vi "MainPr(Calculation)-40.vi"() -> ()   [LabVIEW 2013]
doc: "Main Program for Tracking\nThis VI Represents Front Panel and Control Buttons for Perform Tracking\nPlease, optimize the front panel for your own monitor resolution and needs"
uses:
  <vilib>/vision/Avi.llb/IMAQ AVI2 Refnum.ctl
  <vilib>/vision/NI_Vision_Development_Module.lvlib
panel:
  out "error out":errorcluster
  in  "STOP Program":bool
  in  "Front Panel":T1(tab)
  in  "FrameCtl":u32 max=299
  out "1st Movie (Comparison)":T2(plugin-control)
  out "1st Movie":T2(plugin-control)
  in  "Gamma":sgl format="%.2f"
  in  "Operator G Correction":T3(ring)
  in  "Parameter LoG":sgl format="%.2f"
  in  "Operator LoG":T3(ring)
  in  "1/2 Channels":bool
  in  "Sigma":dbl min=0.1
  in  "FrameCtl2":u32 max=499
  in  "Gray or Binarized?":bool
  out "1st Movie Original":T2(plugin-control)
  out "1st Movie Processed":T2(plugin-control)
  in  "Index for thresholding":i8 min=-9
  in  "Keep Nega-\ntive Values?":bool
  out "Detection Progress":u8(slide) scale=0.0..100.0
  in  "# of Frame":u32 max=499
  in  "Save pics (ex)":bool
  in  "Find ALL objects":bool
  out "Results on 1st Movie":T2(plugin-control)
  out "1st Filtering":T2(plugin-control)
  in  "Try my filters!":bool
  in  "# Erosion":i32=2
  in  "Connectivity":bool=TRUE
  in  "Min  Diam":dbl
  in  "Max  Diam":dbl min=12.0
  in  "Filter Tracks":bool
  out "Tracking progress":u8(slide) scale=0.0..100.0
  in  "Save pictures":bool
  in  "Save movies":bool
  in  "Frame":u32 max=499
  in  "Delete Tracs":bool
  out "1st Filtered":T2(plugin-control)
  in  "dR max":dbl min=1.0
  out "1st Filtering (NN)":T2(plugin-control)
  in  "dR min":dbl min=0.0 max=10.0
  out "Raw #":i32
  out "Saved #":i32
  in  "Tracking Procedure":bool
  in  "Min TRK L":i32 min=2 max=498 step=1
  in  "Closing gaps":i32 min=1 max=498 step=1
  in  "% linearity":i32 min=1 max=100 step=1
  in  "Max angle":dbl min=0.0 max=89.0 step=1.0
  in  "FPS":u32
  in  "FPS Gr":u32
  in  "Save videos \nbelow as *avi":bool
  in  "Save pics below":bool
  in  "Testing Frame":u32 max=17
  out "After Resolving Correspondence Problem":T2(plugin-control)
  out "Connected and Grouped Tracks":T2(plugin-control)
  in  "Tracks group":i32 min=0 max=394
  in  "Save Tracks in Columns (x,y,dx,dy)":bool
  in  "Save Duration of Tracks":bool
  in  "Save Mean Velocities":bool
  out "Duration of Tracks":T4(graph)
  out "Mean Instant Velocities for Each Track":T4(graph)
  in  "Show Distributions":bool
  out "All Path Vels":T4(graph)
  out "All Instant Vels":T4(graph)
  out "mean Instant Vel":dbl format="%#_1f"
  out "StD Instant":dbl format="%#_1g"
  out "mean Path Vel":dbl format="%.1f"
  out "StD Path":dbl format="%.1f"
  in  "Bins":i32=10
  in  "Save All Instant Vels":bool
  in  "Save Path Velocities":bool
  # "Two channels"
  # "*Planning develop-\nment switcher (old)"
  # "One channel"
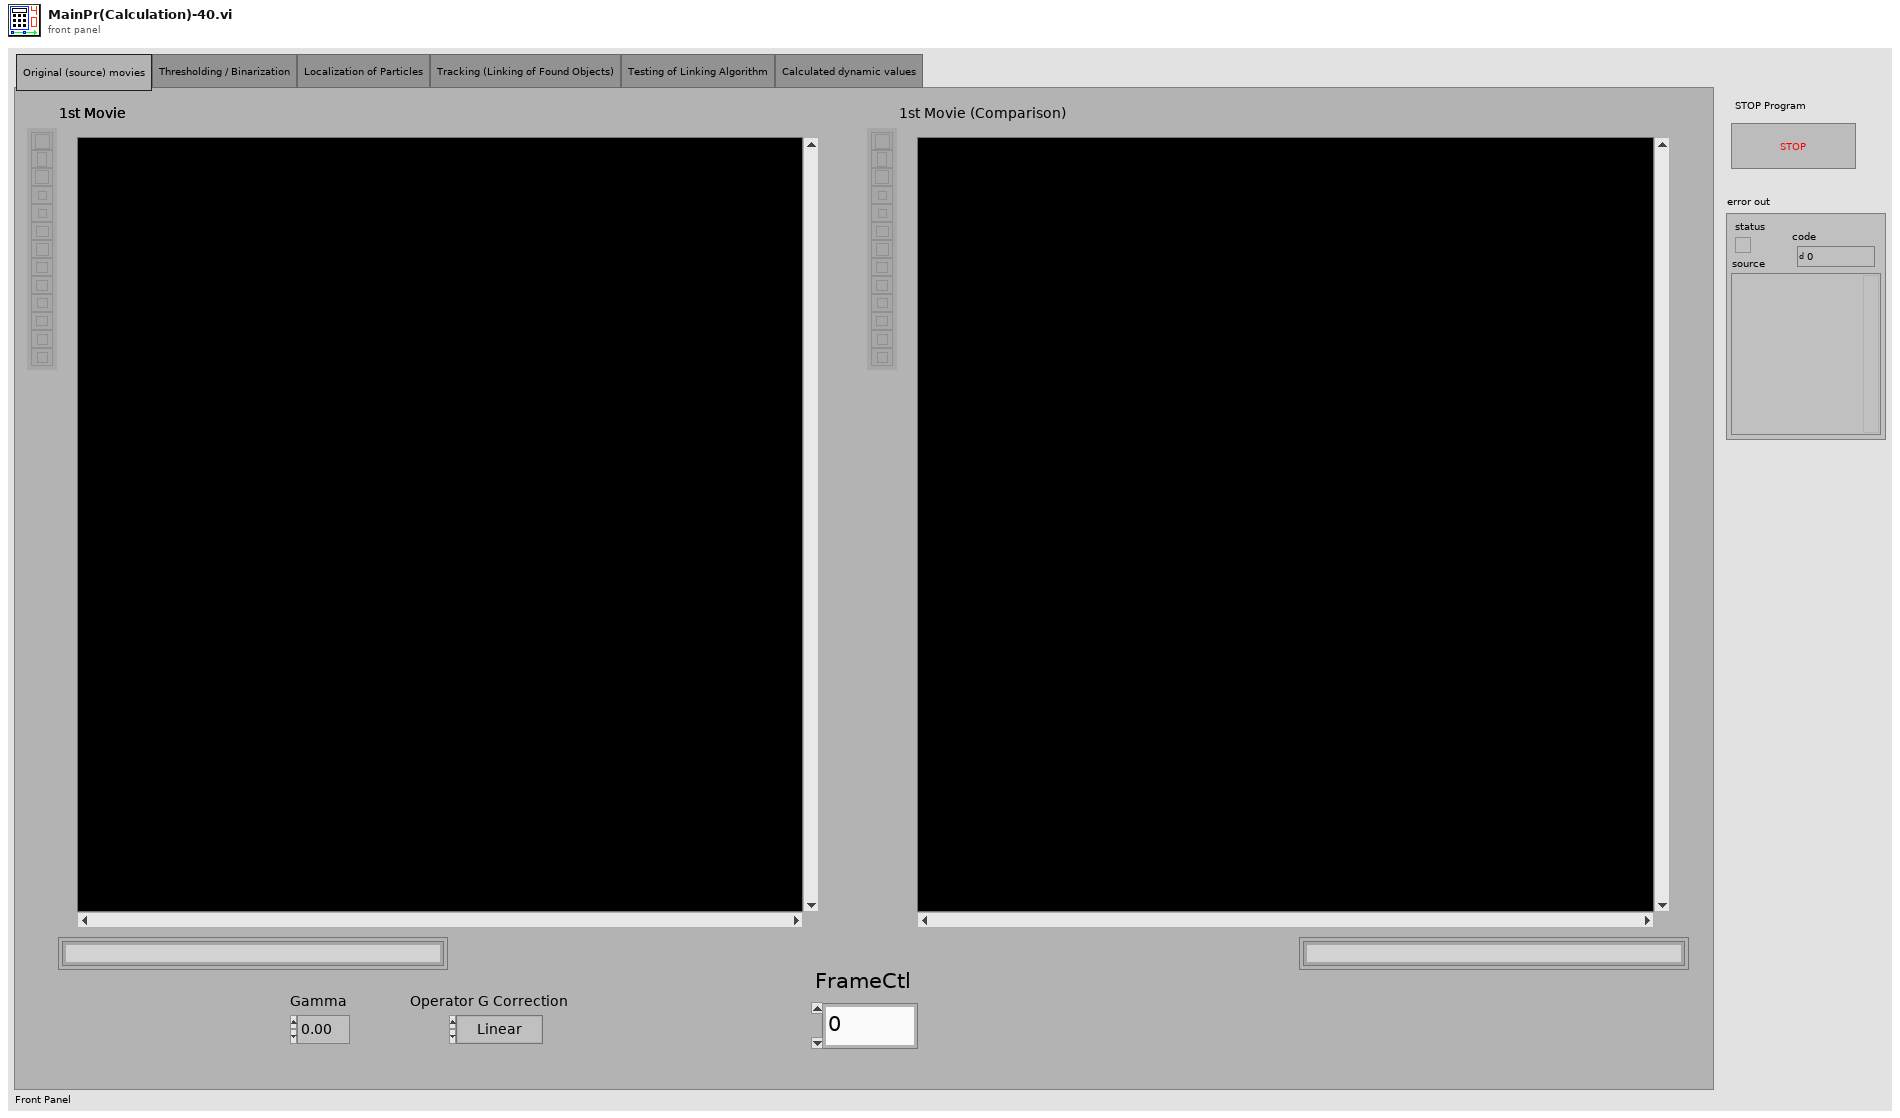
[diagram p1: front panel]
types:
  T1 = enum32{"Original (source) movies", "Thresholding / Binarization", "Localization of Particles", "Tracking (Linking of Found Objects)", "Testing of Linking Algorithm", "Calculated dynamic values"}
  T2 = typedef "IMAQ Image.ctl" = refnum<image>
  T3 = enum32{"Linear", "Log", "Exp", "Square", "Square root", "Power X", "Power 1/X"}
  T4 = cluster{"X Values":dbl[], "Histogram: h(x)":i32[]}
  T5 = typedef "IMAQ AVI2 Refnum.ctl" = refnum<k20>
  T6 = typedef "Image Type" = u32
  T7 = typedef "Particle Parameters" = i32
  T8 = cluster{"[IN] AVI Refnum":T5, "[IN] Image Type":T6, "[IN] Particle Filter Setups":cluster{"Erosion":i32, "Connectivity ":bool, "Type of particle filter":cluster{"Measurement Parameter":T7, "Min  Diam":dbl, "Max  Diam":dbl, "Range":bool, "Range":bool}[]}, "[IN] # Channel":u8, "[IN] Keep Nega-\ntive Values?":bool, "[IN] Image Filtering Settings":cluster{"Gamma Origin":sgl, "Operator Origin":enum32{"Linear", "Log", "Exp", "Square", "Square root", "Power X", "Power 1/X"}, "Gamma LoG":sgl, "Operator LoG":enum32{"Linear", "Log", "Exp", "Square", "Square root", "Power X", "Power 1/X"}, "Sigma":dbl, "Thresholding Index":i8}, "[IN] Binarization Settings":cluster{"MinBin2":sgl, "MaxBin2":sgl}[]}
  T9 = enum8{"Enabled", "Disabled", "Disabled and Grayed Out"}
  T10 = cluster{"dR min ":dbl, "dR max ":dbl, "Closing gaps":i32, "Min TRK L":i32, "% linearity":i32, "Max angle":dbl, "Tracking progress":refnum<vi>}
  T11 = cluster{"X,Y":dbl[][], "Areas particles":dbl[][], "Particle Fil Setups":cluster{"Erosion":i32, "Connectivity ":bool, "Type of particle filter":cluster{"Measurement Parameter":T7, "Min  Diam":dbl, "Max  Diam":dbl, "Range":bool, "Range":bool}[]}, "Tracks, Coordinates":cluster{"(X,Y) Unmoved":dbl[][], "(X,Y,dX,dY) Dur 1 Frame":dbl[][], "(X,Y,dX,dY) W/t Problems":dbl[][], "(X,Y,dX,dY) NN filtered":dbl[][], "(X,Y,dX,dY) TH filtered":dbl[][], "Tracks":cluster{"Tracks":dbl[], "Start Pos":i32}[], "Tracks w/t Problems":cluster{"Tracks":dbl[], "Start Pos":i32}[]}}
  T12 = cluster{"Before Grouped Tracks":cluster{"Tracks":dbl[][], "Start Pos":i32[], "Dot Statuses":i16[][]}[], "After Grouped Tracks":cluster{"Tracks":dbl[][], "Start Pos":i32[], "Dot Statuses":i16[][]}[], "Current\nGroup":i32}
  T13 = cluster{"Gamma Origin":sgl, "Operator Origin":enum32{"Linear", "Log", "Exp", "Square", "Square root", "Power X", "Power 1/X"}, "Gamma LoG":sgl, "Operator LoG":enum32{"Linear", "Log", "Exp", "Square", "Square root", "Power X", "Power 1/X"}, "Sigma":dbl, "Thresholding Index":i8}
  T14 = cluster{"Instant Velocities (All)":dbl[], "Path Velocities (All) ":dbl[], "Tracks in columns":dbl[][], "Mean Instant Velo\ncities for Tracks":dbl[], "MSD":dbl[], "Track duration in frames":u16[], "Track length in pixels":dbl[]}
  T15 = cluster{"Starting Value":sgl, "Incremental Value":sgl, "Histogram":u32[]}
  T16 = cluster{"Erosion":i32, "Connectivity ":bool, "Type of particle filter":cluster{"Measurement Parameter":T7, "Min  Diam":dbl, "Max  Diam":dbl, "Range":bool, "Range":bool}[]}
  T17 = cluster{"Measurement Parameter":T7, "Min  Diam":dbl, "Max  Diam":dbl, "Range":bool, "Range":bool}[]
  T18 = cluster{"Tracks W/T Problems":dbl[], "Start Pos":i32}[]
  T19 = cluster{"All Instant Vel-s":cluster{"X Values":dbl[], "Histogram: h(x)":i32[]}, "mean":dbl, "standard deviation":dbl, "All Path Vel-s":cluster{"X Values":dbl[], "Histogram: h(x)":i32[]}, "mean":dbl, "standard deviation":dbl, "Mean Instan Vel-s":cluster{"X Values":dbl[], "Histogram: h(x)":i32[]}, "mean":dbl, "standard deviation":dbl, "Duration of tracks":cluster{"X Values":dbl[], "Histogram: h(x)":i32[]}, "mean":dbl, "standard deviation":dbl}
  T20 = cluster{"(X,Y) Unmoved":dbl[][], "(X,Y,dX,dY) Dur 1 Frame":dbl[][], "(X,Y,dX,dY) W/t Problems":dbl[][], "(X,Y,dX,dY) NN filtered":dbl[][], "(X,Y,dX,dY) TH filtered":dbl[][], "Tracks":cluster{"Tracks":dbl[], "Start Pos":i32}[], "Tracks w/t Problems":cluster{"Tracks":dbl[], "Start Pos":i32}[]}
  T21 = cluster{"Tracks":dbl[][], "Start Pos":i32[], "Dot Statuses":i16[][]}[]
  T22 = cluster{"[IN] Grouped Tracks":cluster{"Tracks":dbl[][], "Start Pos":i32[], "Dot Statuses":i16[][]}[], "[IN] Tracks group":i32, "[IN] Testing Frame ":u32}
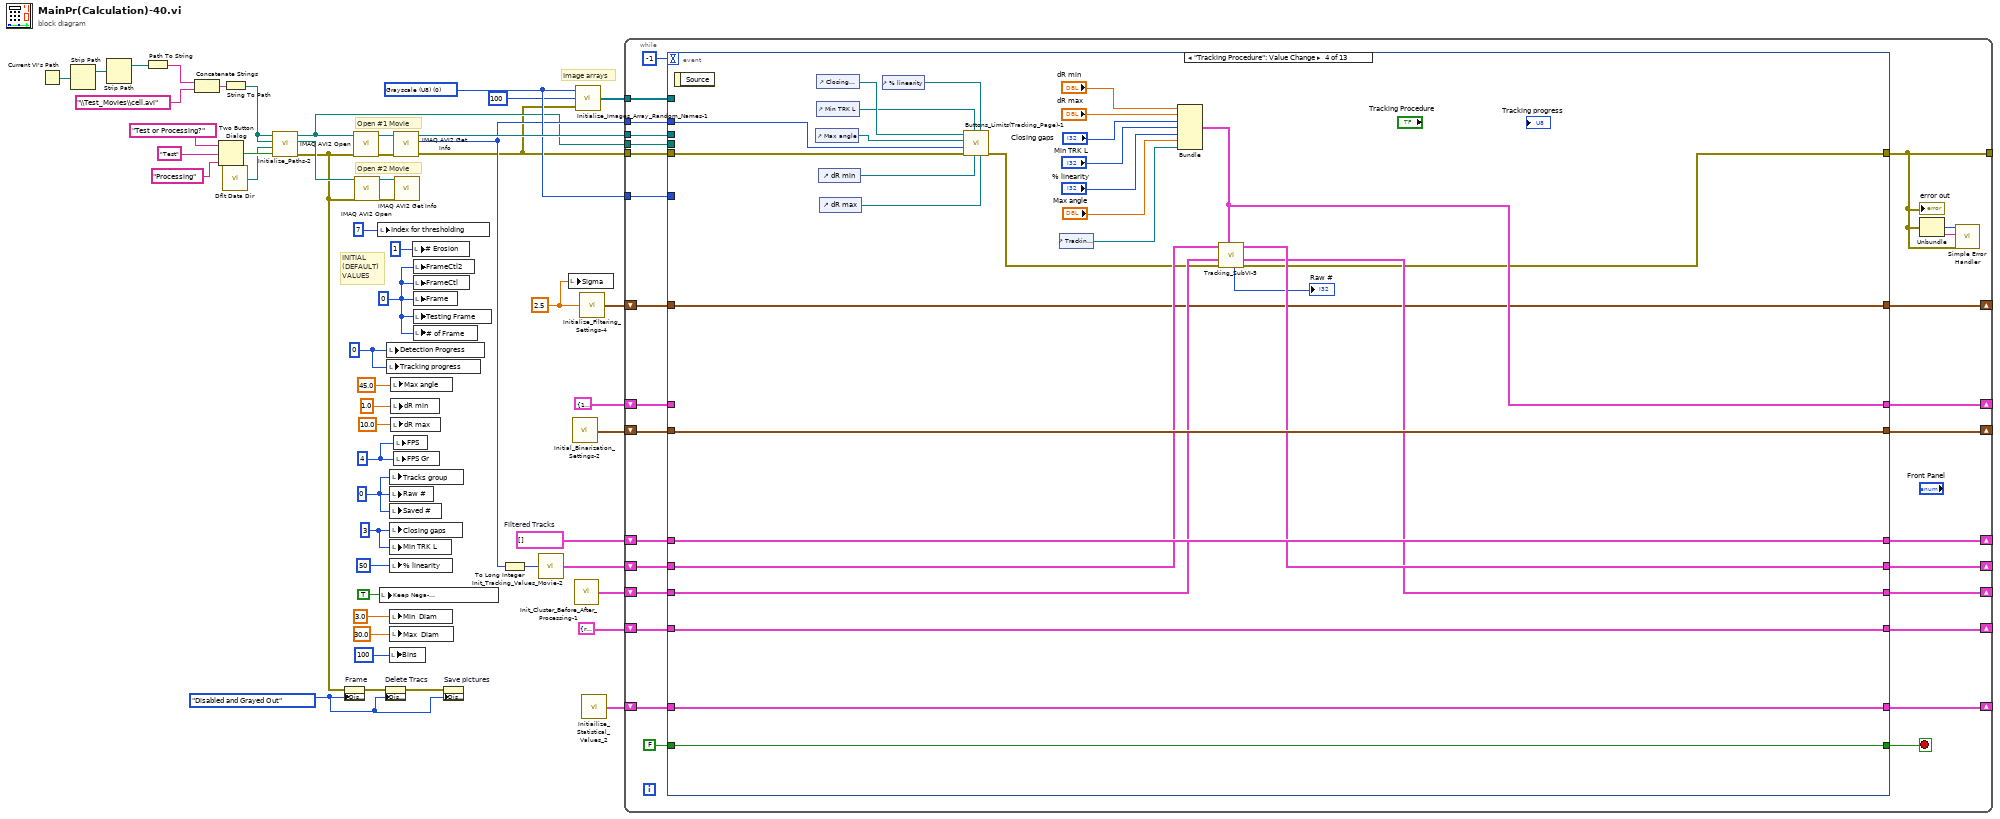
[diagram p0: block diagram]
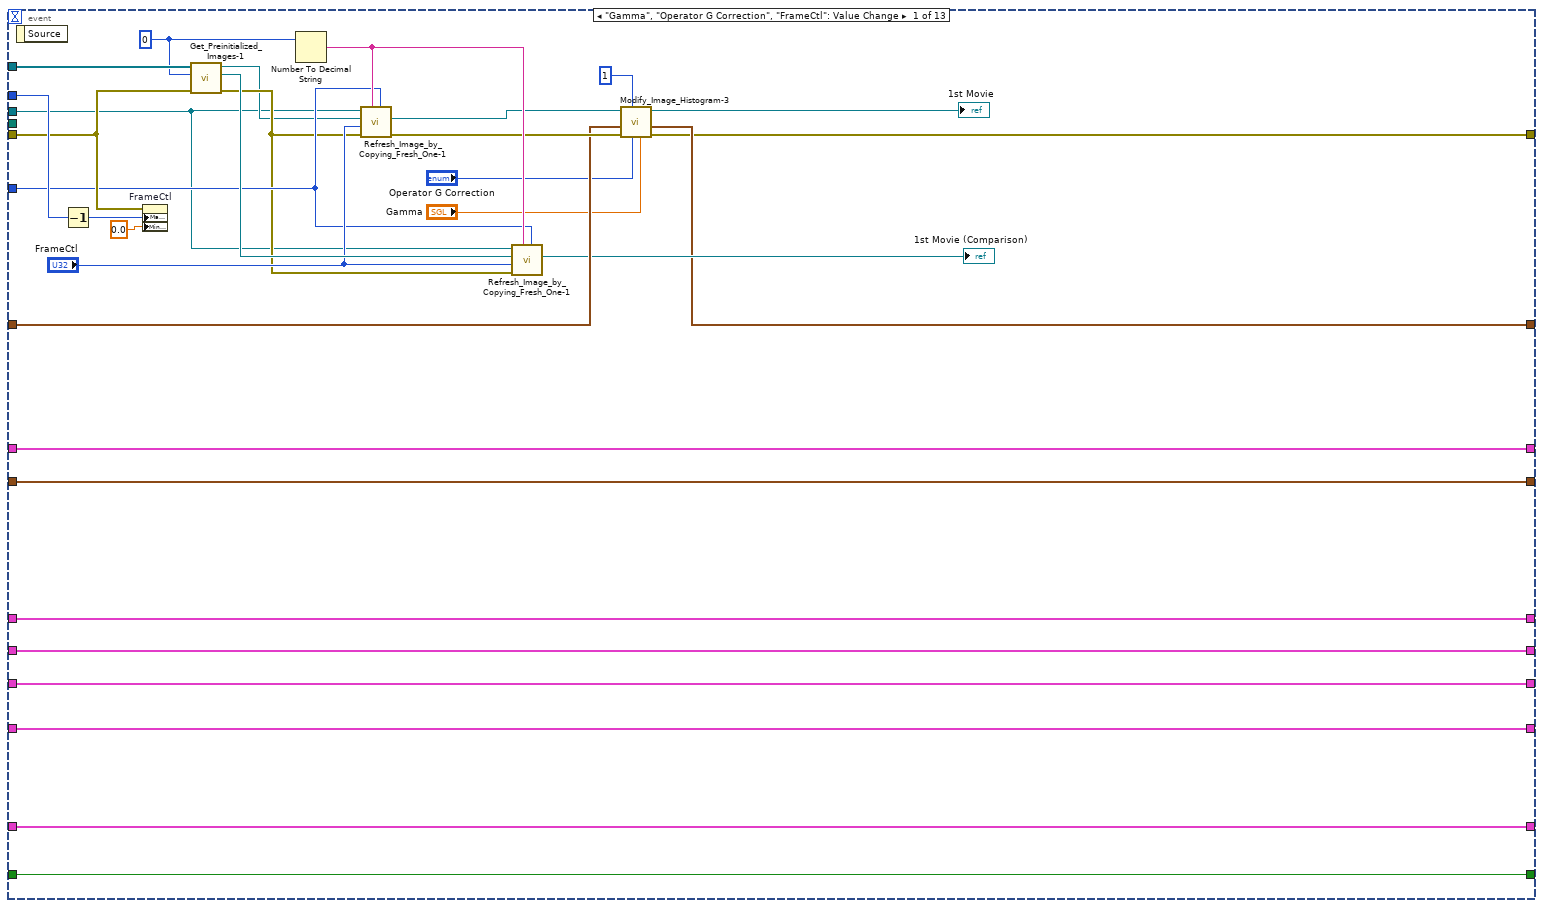
[diagram p2: hidden frame]
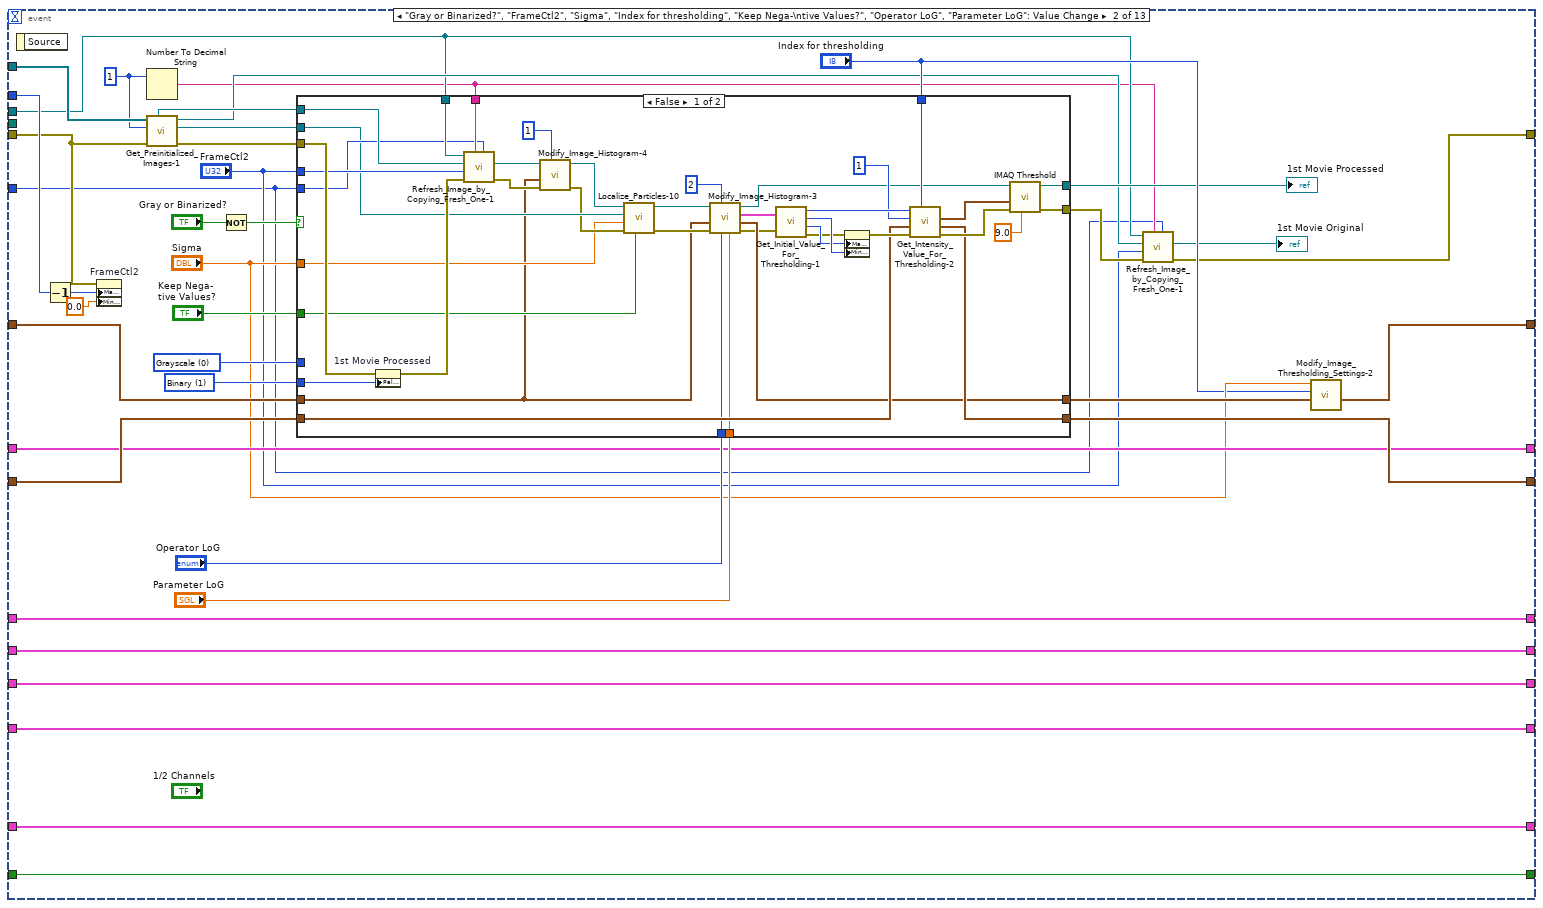
[diagram p3: hidden frame]
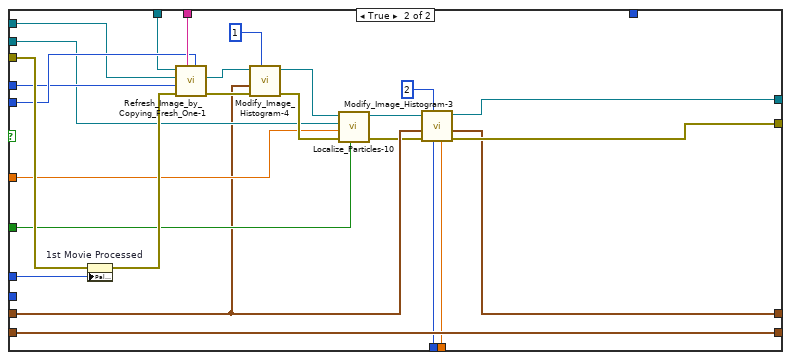
[diagram p4: hidden frame]
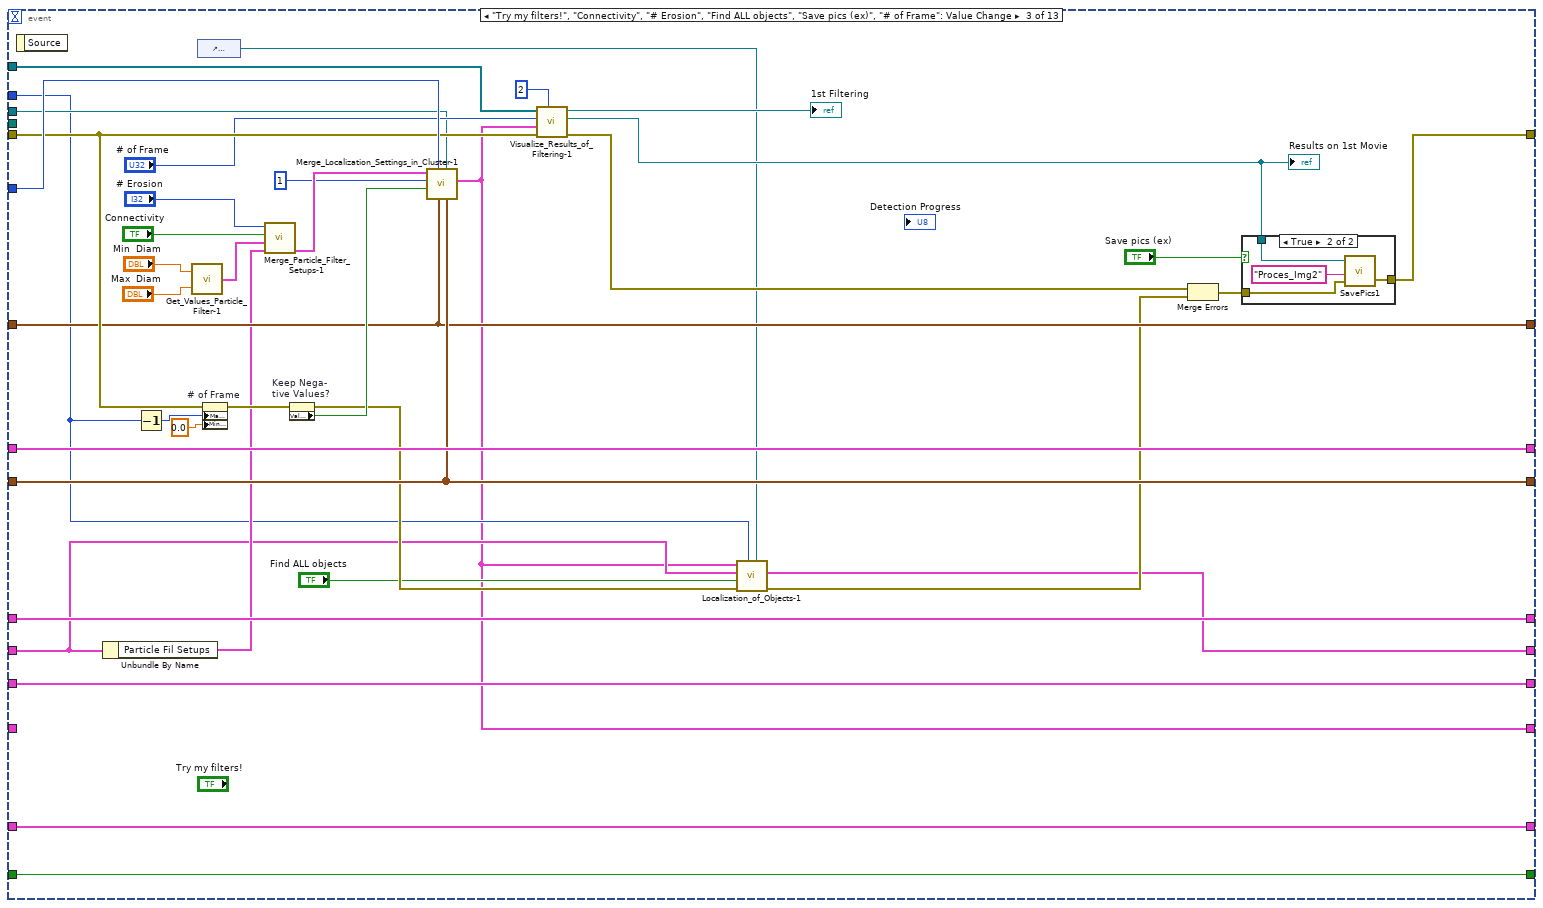
[diagram p5: hidden frame]
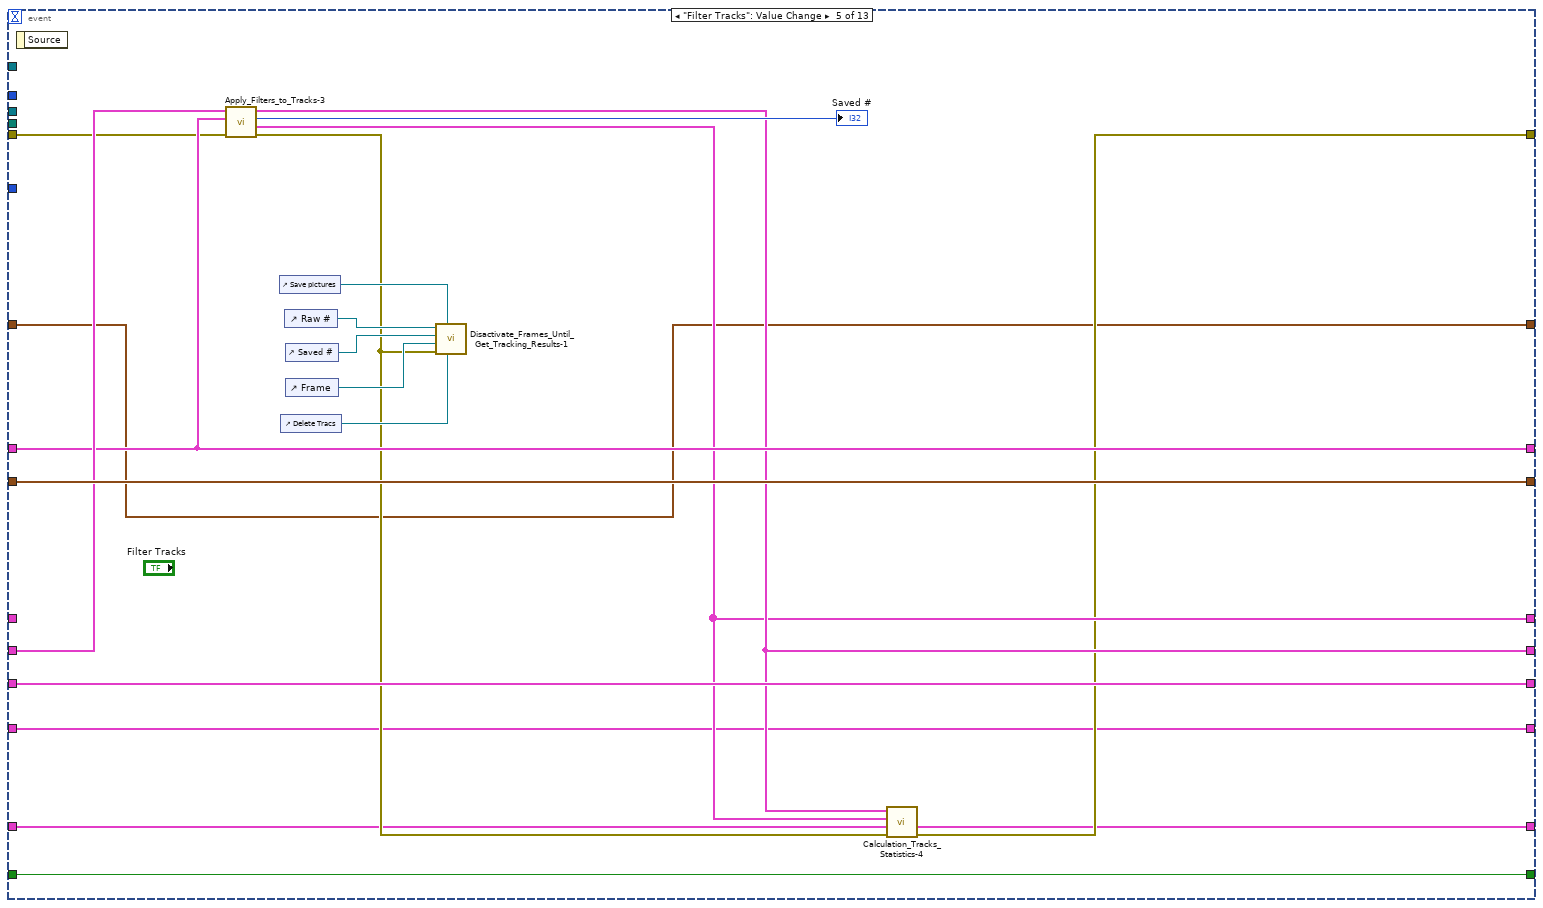
[diagram p7: hidden frame]
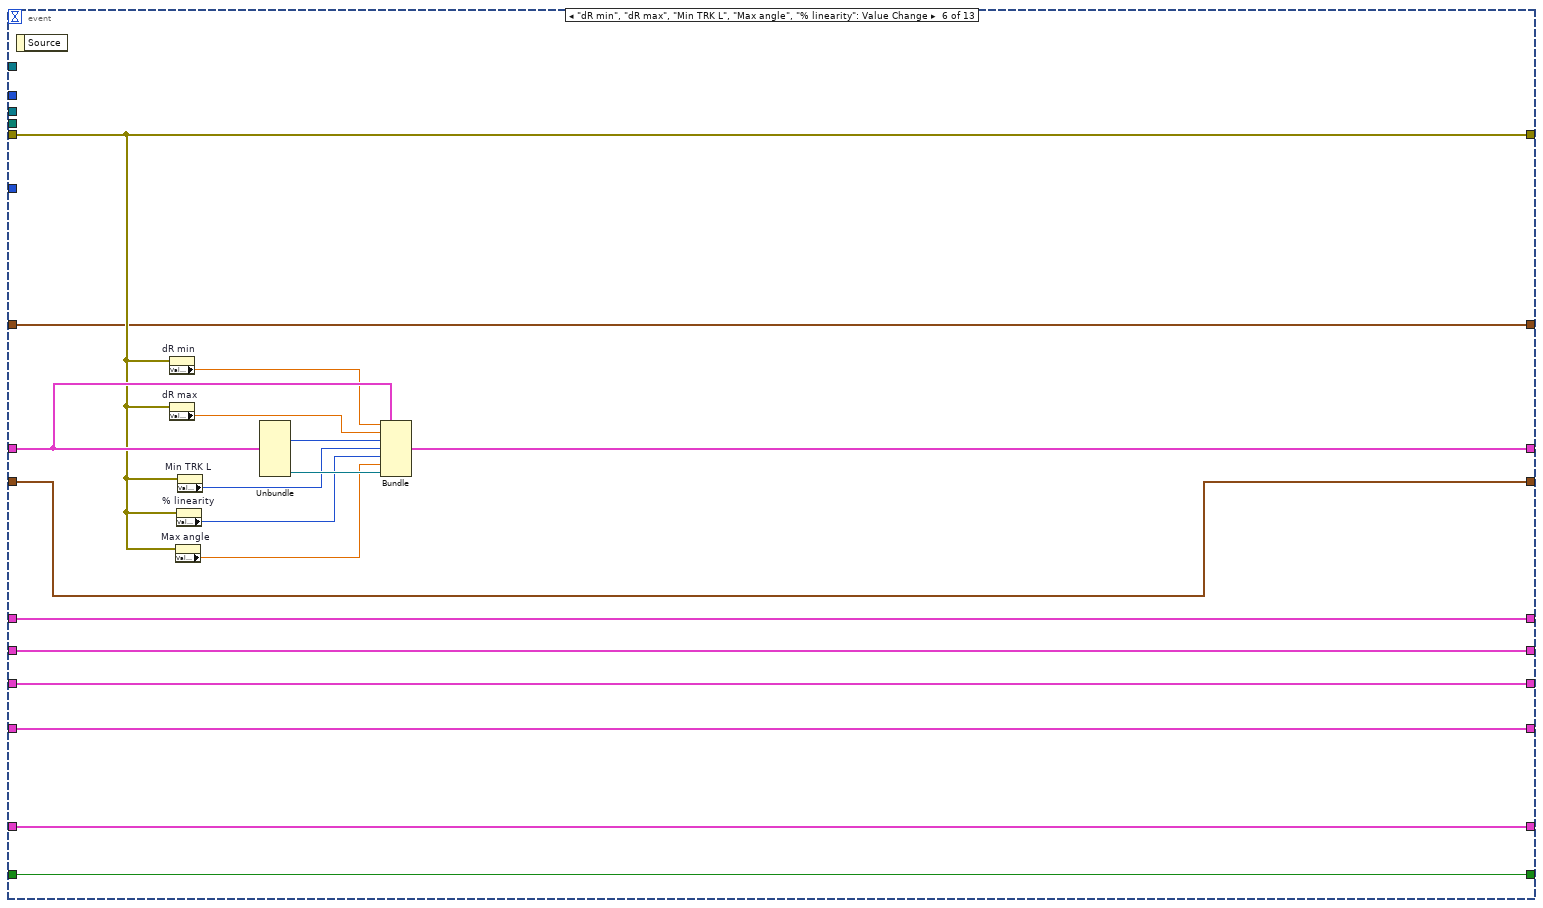
[diagram p8: hidden frame]
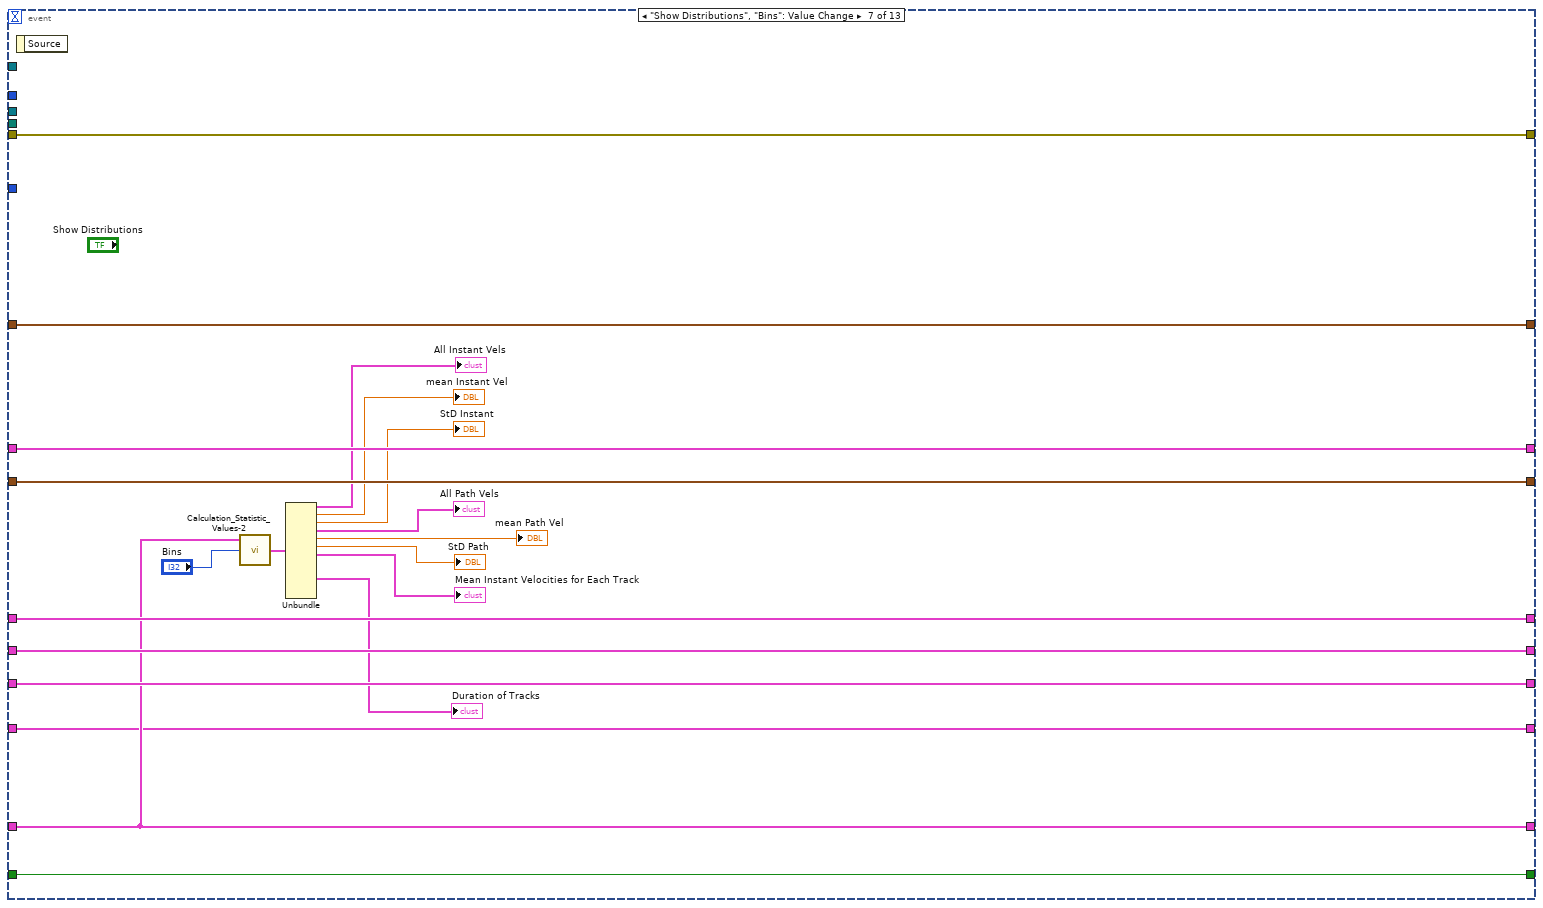
[diagram p9: hidden frame]
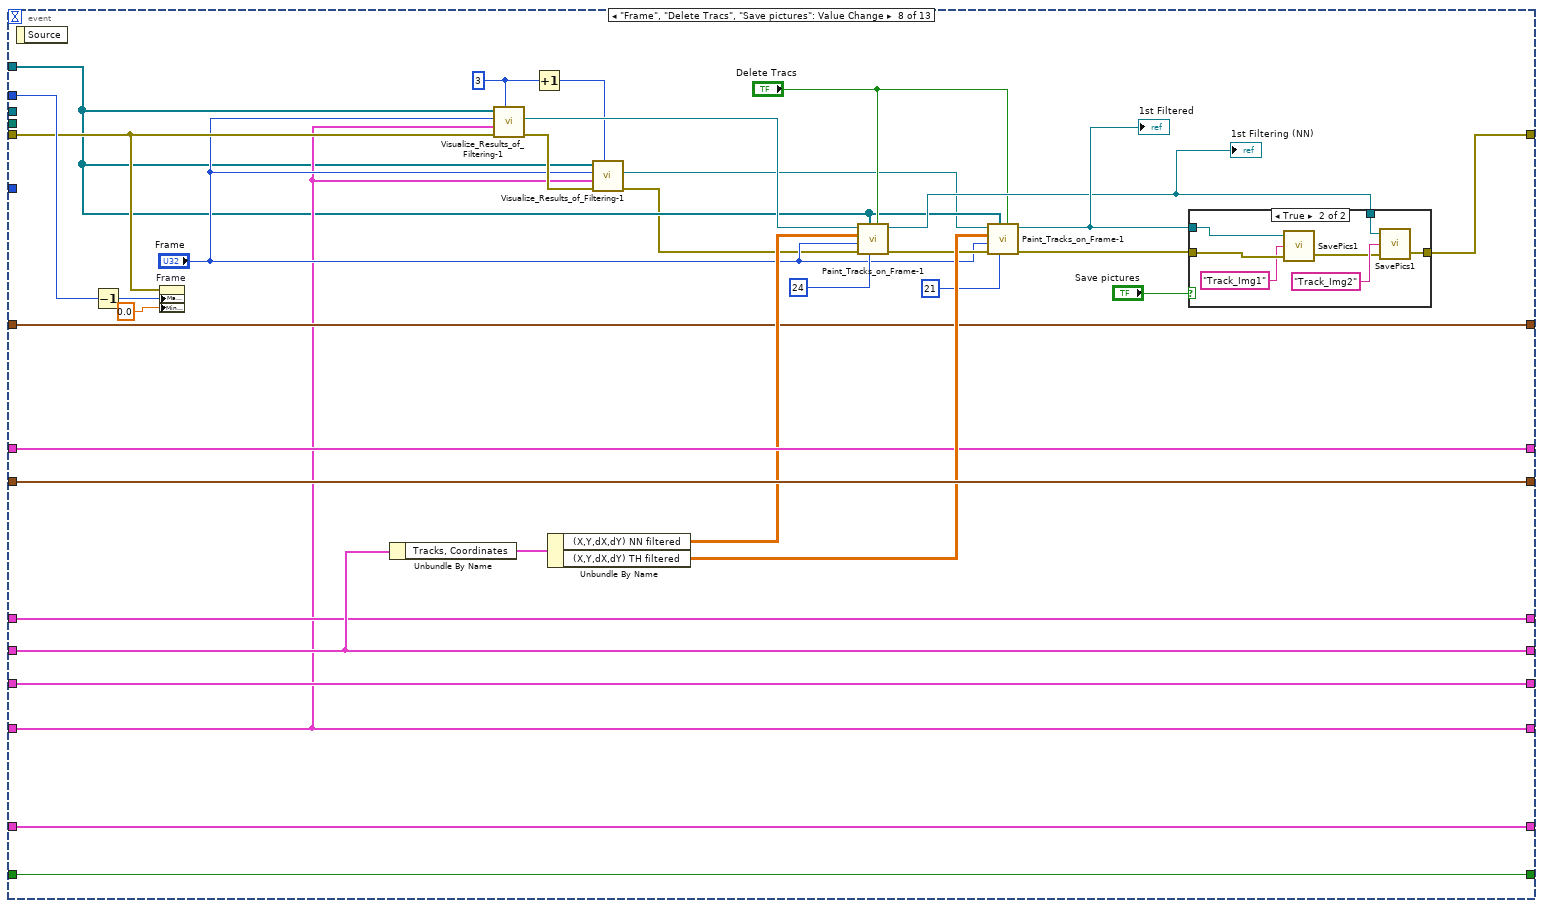
[diagram p10: hidden frame]
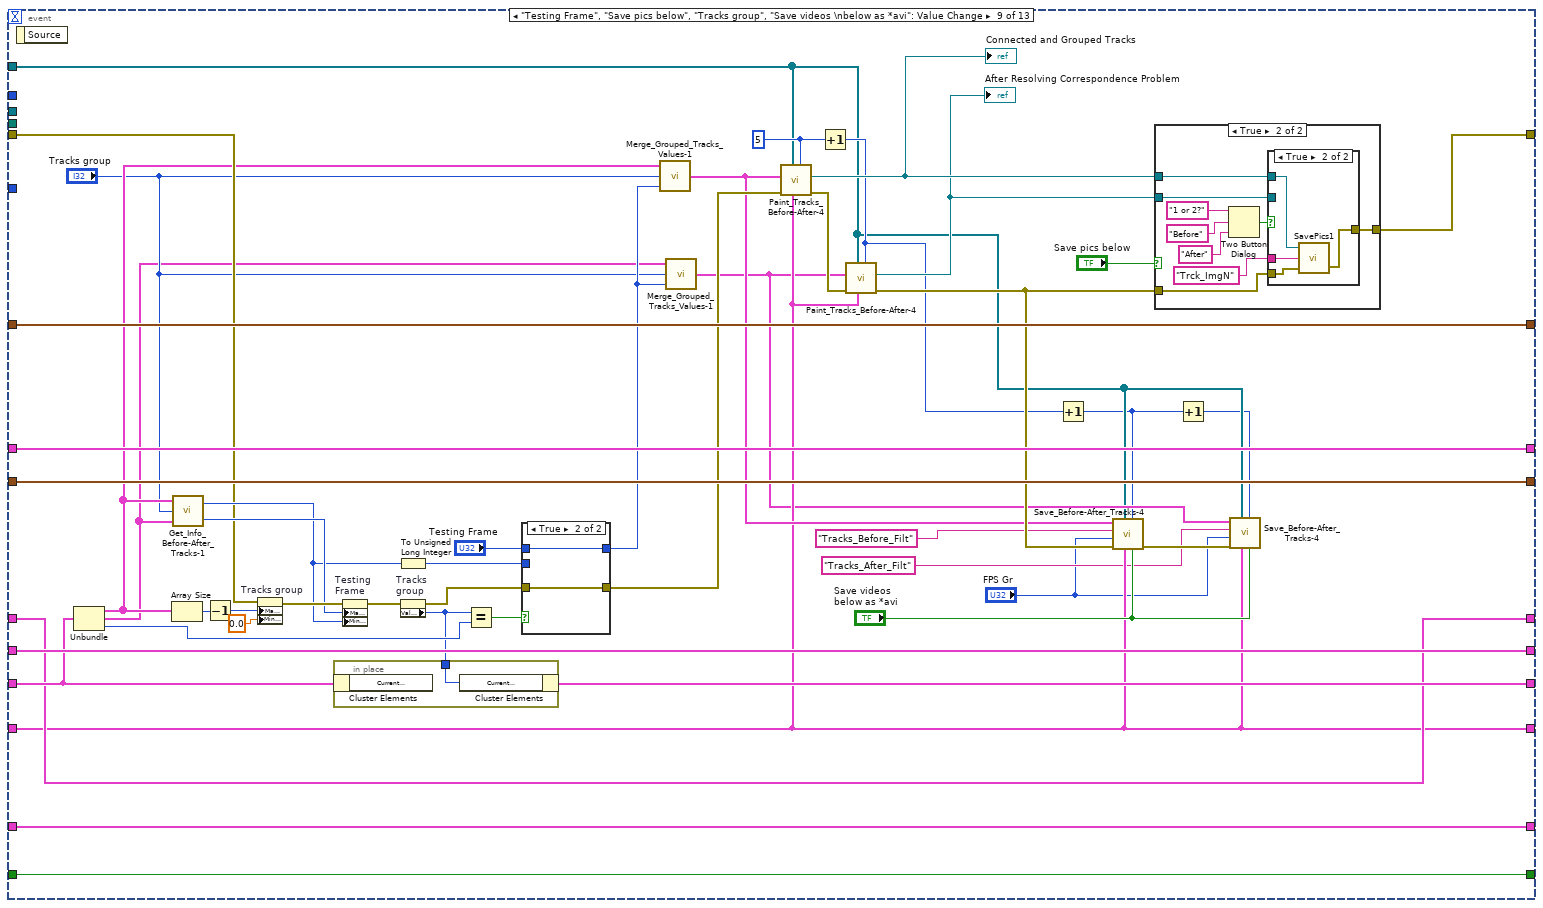
[diagram p12: hidden frame]
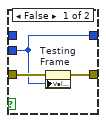
[diagram p13: hidden frame]
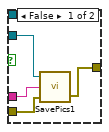
[diagram p15: hidden frame]
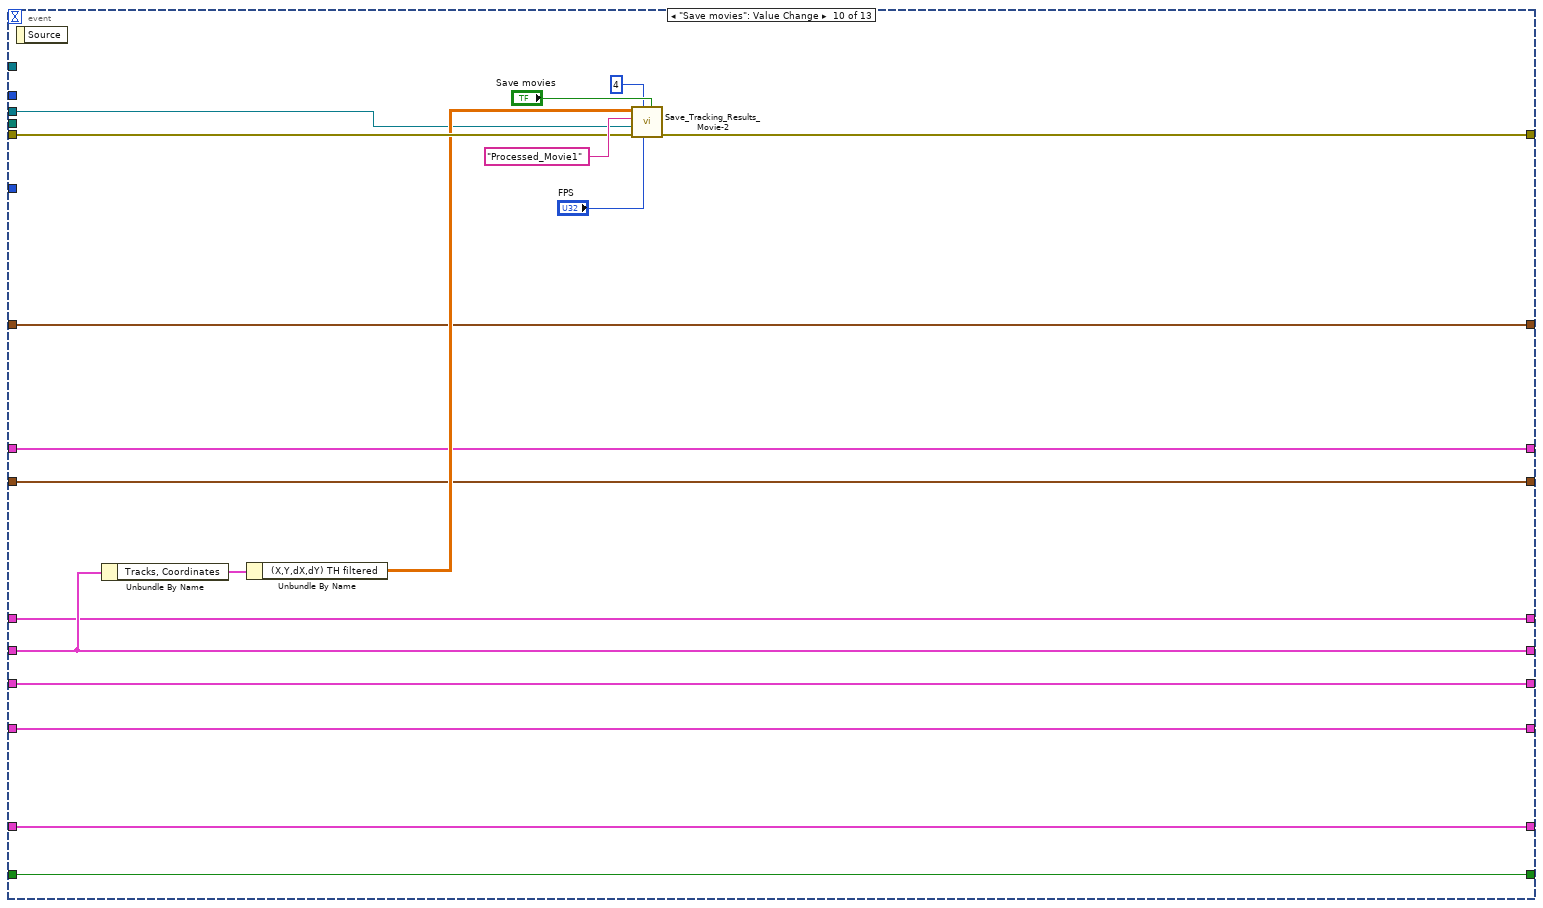
[diagram p16: hidden frame]
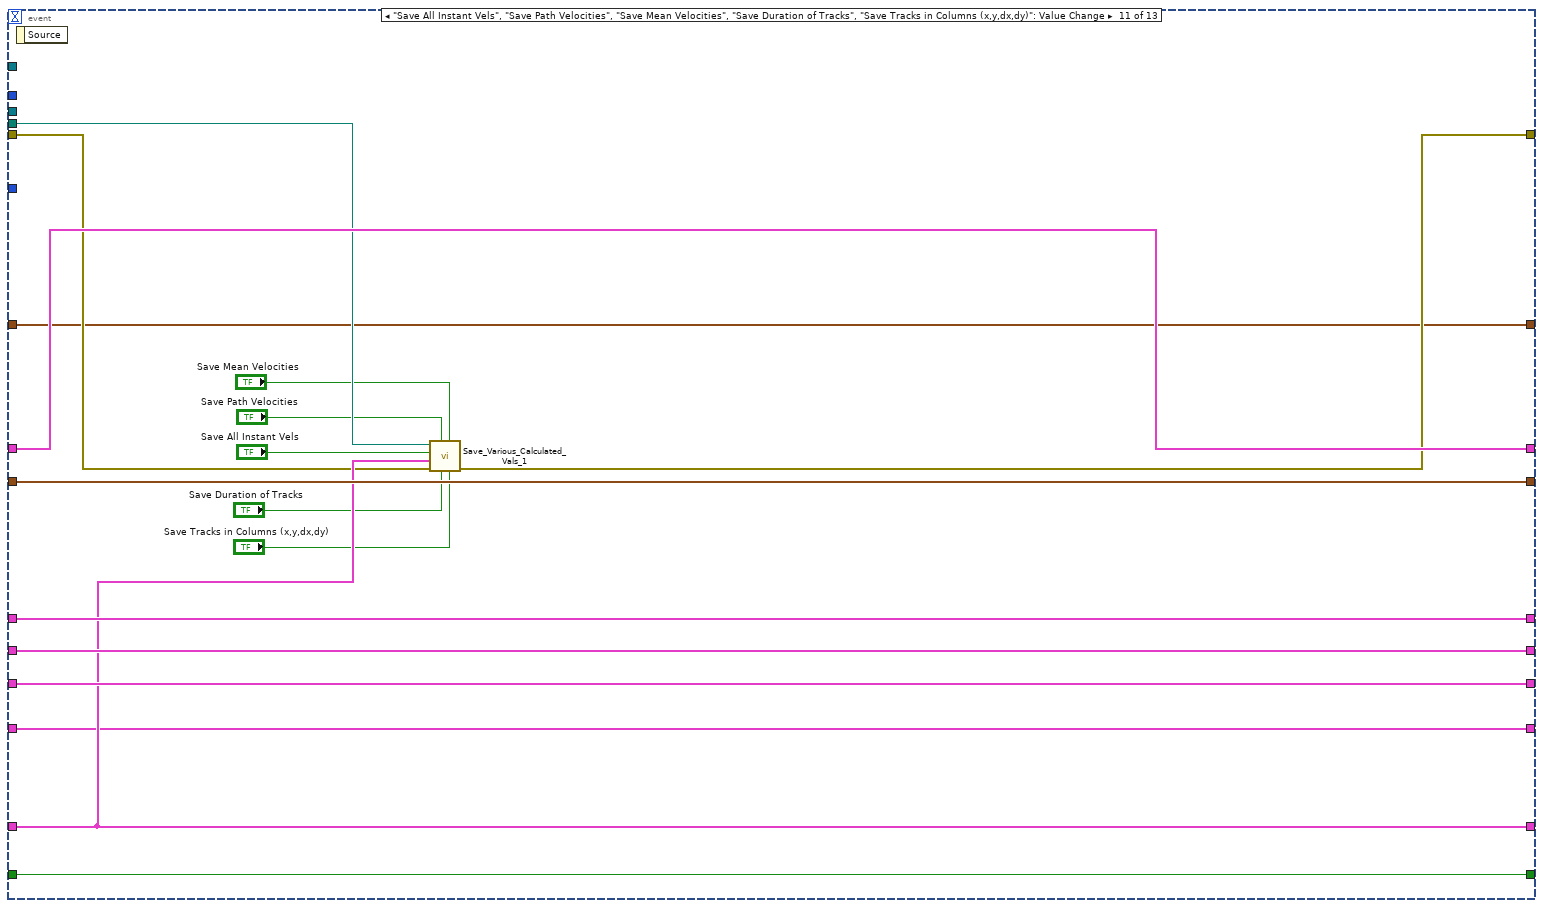
[diagram p17: hidden frame]
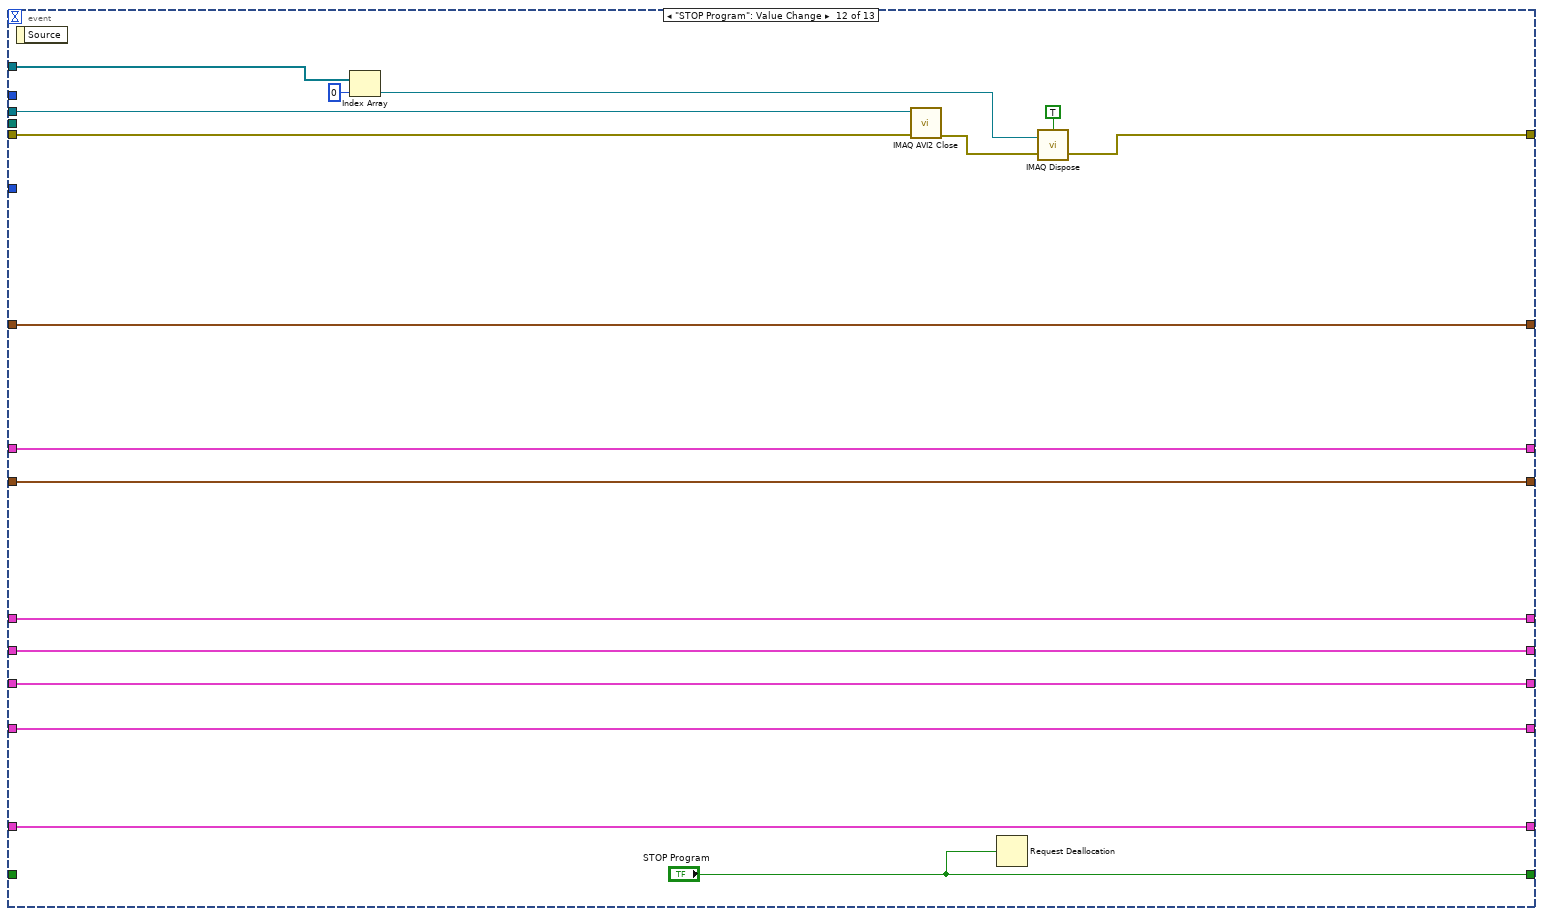
[diagram p18: hidden frame]
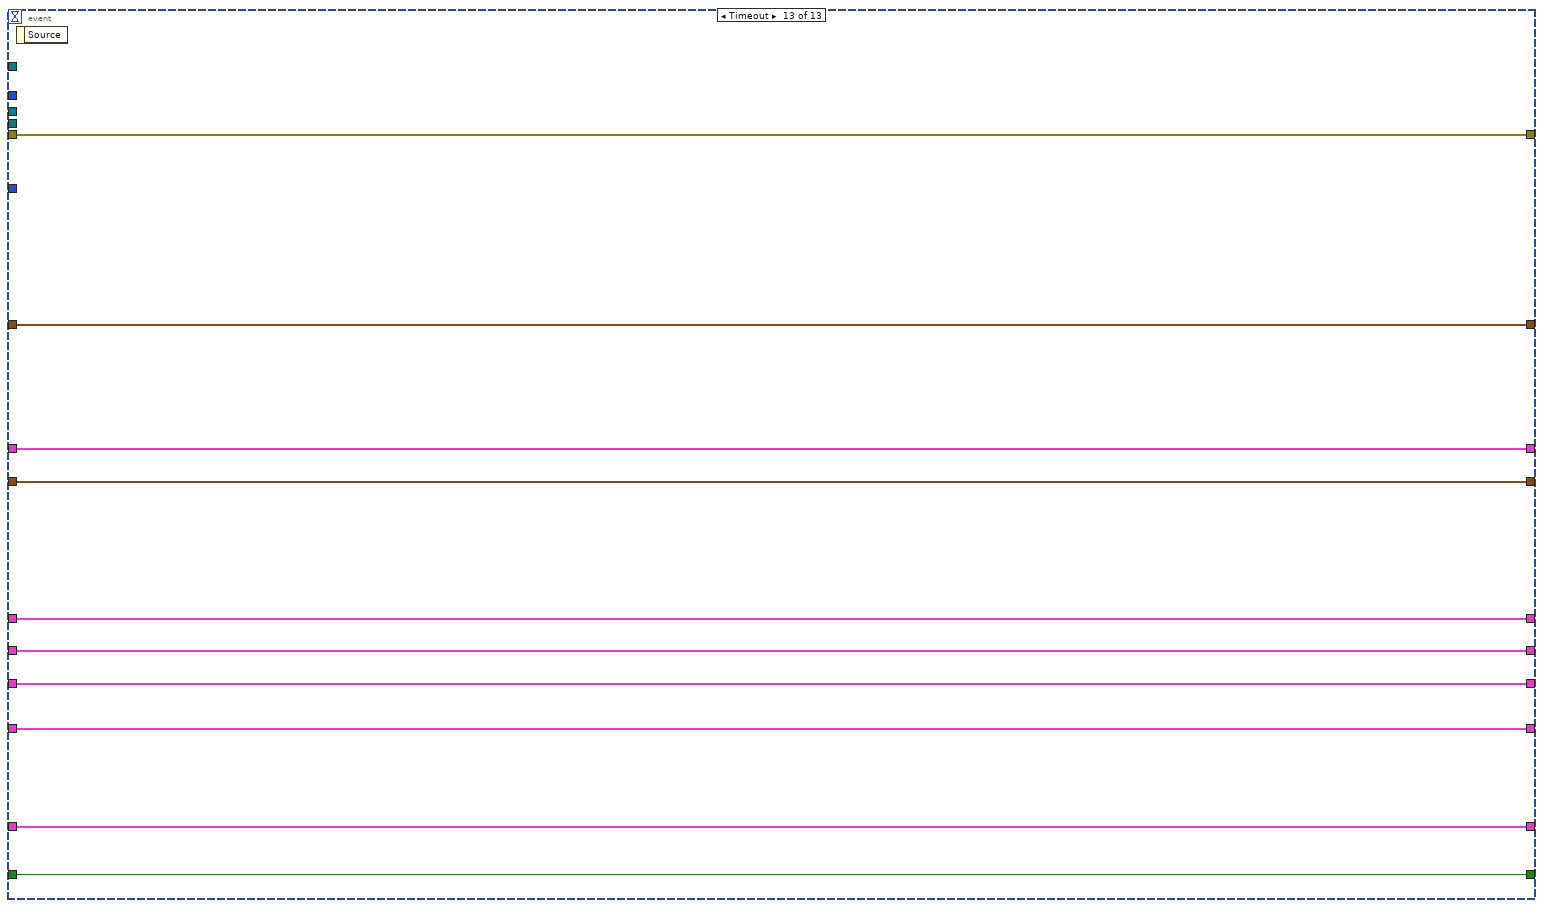
[diagram p19: hidden frame]
diagram:
  w7 = 0 ("Tracks group")
  w9 = u32 4 ("FPS")
  w22 = cluster{"Tracks":dbl[], "Start Pos":i32}[] []  # Filtered Tracks
  w23 = T9."Disabled and Grayed Out" ("Disabled")
  w12 = u32 0 ("Testing Frame")
  w14 = u8 0 ("Progress")
  w16 = 2.5 ("Sigma")
  w6 = 3 ("Closing gaps")
  w44 = T6 0 items=["Grayscale (U8)", "Grayscale (I16)", "Grayscale (SGL)", "Complex (CSG)", "RGB (U32)", "HSL (U32)", "RGB (U64)", "Grayscale (U16)"] ("Image Type")
  # "INITIAL\n(DEFAULT)\nVALUES"
  # "Image arrays"
  # "Open #2 Movie"
  # "Open #1 Movie"
  n1 = Current VI's Path() -> (path=w32:path)
  n2 = Strip Path(path=w32) -> (stripped path=w30:path)  [unwired: 1 out]
  n3 = Strip Path(path=w30) -> (stripped path=w29:path)  [unwired: 1 out]
  n4 = Path To String(path=w29) -> (string=w37:string)
  n5 = Concatenate Strings(w37, "\\Test_Movies\\cell.avi" ("string")) -> (w34:string)
  n6 = Two Button Dialog(message="Test or Processing?", 1:"Processing" ("F button name (\"Cancel\")"), 2:"Test" ("T button name (\"OK\")")) -> (T button?=w40:bool)
  n7 = call <vilib>:"Dflt Data Dir.vi"() -> ("App:Default Data Directory"=w35:path)
  n8 = String To Path(string=w34) -> (path=w33:path)
  n9 = call "Initialize_Paths-2.vi"("Test or Processing?"=w40, "start path"=w35, "AVI File Path #2"=w33, "AVI File Path #1"=w33) -> ("ERROR OUT"=w17:errorcluster, "AVI File Path #2 OUT"=w39:path, "AVI File Path #1 OUT"=w31:path)  [unwired: 1 out]
  n10 = property on="Frame" class="DigNum (strict)"(error in=w17, "DisabledEnum"=w23) -> (error out=w25:errorcluster)  [unwired: 1 in, 1 out]
  n11 = call "IMAQ AVI2 Open"("error in (no error)"=w17, "AVI File Path"=w31) -> ("error out"=w52:errorcluster, "AVI Refnum"=w53:T5)  [unwired: 8 in]
  n12 = call "IMAQ AVI2 Open"("error in (no error)"=w17, "AVI File Path"=w39) -> ("error out"=w51:errorcluster, "AVI Refnum"=w50:T5)  [unwired: 8 in]
  n13 = local write "Index for thresholding"(i8 7 ("Index for \nthresholding")) -> ()
  n14 = local write "Keep Nega-\ntive Values?"(TRUE ("Keep Nega-\ntive Values?")) -> ()
  n15 = property on="Delete Tracs" class="Bool"(error in=w25, "DisabledEnum"=w23) -> (error out=w24:errorcluster)  [unwired: 1 in, 1 out]
  n16 = local write "Detection Progress"(w14) -> ()
  n17 = local write "Tracking progress"(w14) -> ()
  n18 = local write "Bins"(100 ("Intervals")) -> ()
  n19 = local write "Tracks group"(w7) -> ()
  n20 = local write "Raw #"(w7) -> ()
  n21 = local write "Saved #"(w7) -> ()
  n22 = local write "Closing gaps"(w6) -> ()
  n23 = local write "Min TRK L"(w6) -> ()
  n24 = local write "% linearity"(50 ("% linearity")) -> ()
  n25 = local write "Min  Diam"(3.0 ("Min  Diam")) -> ()
  n26 = local write "Max  Diam"(30.0 ("Max  Diam")) -> ()
  n27 = local write "Max angle"(45.0 ("Max angle")) -> ()
  n28 = local write "dR min"(1.0 ("dR min")) -> ()
  n29 = local write "dR max"(10.0 ("dR max")) -> ()
  n30 = call "IMAQ AVI2 Get Info"("error in (no error)"=w52, "AVI Refnum"=w53) -> ("error out"=w21:errorcluster, "Number of Frames"=w43:u32, "AVI Refnum (duplicate)"=w49:T5)  [unwired: 5 in, 2 out]
  n31 = local write "FPS"(w9) -> ()
  n32 = local write "FPS Gr"(w9) -> ()
  n33 = call "IMAQ AVI2 Get Info"("error in (no error)"=w51, "AVI Refnum"=w50) -> ()  [unwired: 5 in, 5 out]
  n34 = local write "# Erosion"(1 ("# Erosion")) -> ()
  n35 = local write "FrameCtl2"(w12) -> ()
  n36 = local write "FrameCtl"(w12) -> ()
  n37 = local write "Frame"(w12) -> ()
  n38 = local write "Testing Frame"(w12) -> ()
  n39 = local write "# of Frame"(w12) -> ()
  n40 = property on="Save pictures" class="Bool"(error in=w24, "DisabledEnum"=w23) -> ()  [unwired: 1 in, 2 out]
  n41 = To Long Integer(number=w43) -> (32bit integer=w27:i32)
  n42 = call "Init_Tracking_Values_Movie-2.vi"("[IN] # Frames"=w27) -> ("[OUT] Movie Values\n(Empty Cluster)"=w26:T11)
  n43 = local write "Sigma"(w16) -> ()
  n44 = call "Initial_Binarization_Settings-2.vi"() -> ("Binarization Settings"=w45:cluster{"MinBin2":sgl, "MaxBin2":sgl}[])
  n45 = call "Init_Cluster_Before_After_Processing-1.vi"() -> ("[OUT] Before-After"=w38:T12)
  n46 = call "Initialize_Images_Array_Random_Names-1.vi"("error IN"=w21, "# Pics"=100, "Image Type"=w44) -> ("Images Array"=w42:T2[])
  n47 = call "Initialize_Filtering_Settings-4.vi"("Sigma #1"=w16) -> ("[OUT] Image Filtering Settings"=w19:T13)
  n48 = call "Initiailize_Statistical_Values_2.vi"() -> ("Statistics"=w20:T14)
  n49 = while {
    tunnel: w21 -> [w75]
    tunnel: w43 -> [w78]
    tunnel: [w70] -> _
    tunnel: w49 -> [w79]
    shift-right: [w73] -> _
    shift-left: w26 -> [w74]
    shift-right: [w71] -> _
    shift-left: w20 -> [w72]
    shift-right: [w68] -> _
    shift-left: w38 -> [w69]
    shift-right: [w66] -> _
    shift-left: w45 -> [w67]
    tunnel: w44 -> [w65]
    tunnel: w42 -> [w64]
    tunnel: w31 -> [w62]
    shift-right: [w61] -> _
    shift-left: T10 {"dR min "=1.0, "dR max "=10.0, "Closing gaps"=3, "Min TRK L"=3, "% linearity"=50, "Max angle"=46.0, "Tracking progress"=refnum} -> [w60]
    shift-right: [w58] -> _
    shift-left: w22 -> [w59]
    shift-right: [w56] -> _
    shift-left: w19 -> [w57]
    shift-right: [w54] -> _
    shift-left: T8 {"[IN] AVI Refnum"=refnum, "[IN] Image Type"=0, "[IN] Particle Filter Setups"={"Erosion"=0, "Connectivity "=FALSE, "Type of particle filter"=[]}, "[IN] # Channel"=0, "[IN] Keep Nega-\ntive Values?"=FALSE, "[IN] Image Filtering Settings"={"Gamma Origin"=0.0, "Operator Origin"=enum."Linear", "Gamma LoG"=0.0, "Operator LoG"=enum."Linear", "Sigma"=0.0, "Thresholding Index"=0}, "[IN] Binarization Settings"=[]} ("[OUT] Localization Settings") -> [w55]
    stop <- w81 stop-if-true
    n50 = event shown="[3] \"Tracking Procedure\": Value Change" {
      selector: _ -> [_ _ _ _ _ _ _ _ _ _ _ _ _]
      dyn-events: _ -> [_ _ _ _ _ _ _ _ _ _ _ _ _]
      timeout: -1 -> [_ _ _ _ _ _ _ _ _ _ _ _ _]
      tunnel: [w95 w131 w246 w274 w305 w322 w344 w367 w419 w467 w492 "STOP Program" w517] -> w81
      tunnel: w79 -> [w96 w117 w228 _ _ _ _ _ _ w471 _ w506 _]
      tunnel: w75 -> [w105 w141 w234 w289 w300 w316 w348 w358 w412 w474 w486 w505 w522]
      tunnel: w78 -> [w106 w142 w223 w288 _ _ _ w373 _ _ _ _ _]
      tunnel: [w83 w120 w252 w264 w295 w316 w348 w380 w429 w468 w487 w501 w522] -> w70
      tunnel: w74 -> [w112 w146 w219 w271 w302 w325 w346 w379 w434 w477 w495 w512 w521]
      tunnel: [w112 w146 w221 w267 w298 w325 w346 w379 w434 w477 w495 w512 w521] -> w73
      tunnel: w72 -> [w109 w147 w254 w272 w294 w323 w341 w376 w436 w478 w488 w510 w520]
      tunnel: [w109 w147 w254 w272 w293 w323 w341 w376 w436 w478 w488 w510 w520] -> w71
      tunnel: w69 -> [w108 w145 w251 w269 w304 w324 w345 w374 w418 w476 w494 w509 w519]
      tunnel: [w108 w145 w251 w265 w304 w324 w345 w374 w416 w476 w494 w509 w519] -> w68
      tunnel: w67 -> [w107 w144 w237 w290 w303 w314 w347 w372 w420 w469 w493 w508 w518]
      tunnel: [w107 w143 w237 w290 w303 w314 w347 w372 w420 w469 w493 w508 w518] -> w66
      tunnel: w65 -> [w99 w115 w236 _ _ _ _ _ _ _ _ _ _]
      tunnel: w64 -> [w104 w140 w233 _ _ _ _ w351 w393 _ _ w507 _]
      tunnel: FALSE ("STOP Program") -> [w95 w131 w246 w274 w305 w322 w344 w367 w419 w467 w492 _ w517]
      tunnel: w62 -> [_ _ _ _ _ _ _ _ _ _ w485 _ _]
      tunnel: [w94 w130 w245 w270 w301 w313 w343 w366 w415 w466 w491 w500 w516] -> w61
      tunnel: w60 -> [w94 w130 w245 _ w301 w328 w343 w366 w415 w466 w491 w500 w516]
      tunnel: w59 -> [w93 w129 w244 w273 _ w326 w342 w365 w414 w465 w490 w499 w515]
      tunnel: [w93 w129 w244 w273 w297 w326 w342 w365 w414 w465 w490 w499 w515] -> w58
      tunnel: w57 -> [w90 w127 w227 w263 w292 w312 w330 w359 w413 w462 w480 w497 w514]
      tunnel: [w84 w114 w227 w263 w292 w312 w330 w359 w413 w462 w480 w497 w514] -> w56
      tunnel: w55 -> [w82 w113 _ w262 w291 w311 w329 w352 w396 w461 w479 w496 w513]
      tunnel: [w82 w113 w218 w262 w291 w311 w329 w352 w396 w461 w479 w496 w513] -> w54
      event "Gamma", "Operator G Correction", "FrameCtl": Value Change {
        w103 = i8 0 ("[IN] Number of event")
        n51 = event-data() -> ()  [unwired: 1 in, 1 out]
        n52 = Decrement(x=w106) -> (x-1=w110:u32)
        n53 = property on="FrameCtl" class="DigNum (strict)"(error in=w105, "Maximum"=w110, "Minimum"=0.0 ("Data Entry Limits:Minimum")) -> ()  [unwired: 1 in, 2 out]
        n54 = call "Get_Preinitialized_Images-1.vi"("error IN"=w105, "[IN] Number of event"=w103, "[IN] Images Array"=w104) -> ("error OUT"=w98:errorcluster, "[OUT] Processed Image #1"=w102:T2, "[OUT] Source Image #2"=w97:T2)  [unwired: 1 in, 2 out]
        n55 = Number To Decimal String(number=w103) -> (decimal integer string=w100:string)  [unwired: 1 in]
        n56 = call "Refresh_Image_by_Copying_Fresh_One-1.vi"("[IN] Image Type"=w99, "[IN] Unique ID\n(# of Event)"=w100, "error IN"=w98, "Frame Number"="FrameCtl", "[IN] Preinitialized Image"=w97, "[IN] AVI Refnum"=w96) -> ("error OUT"=w91:errorcluster, "[OUT] Frame"=w92:T2)  [unwired: 1 in, 1 out]
        n57 = call "Refresh_Image_by_Copying_Fresh_One-1.vi"("[IN] Image Type"=w99, "[IN] Unique ID\n(# of Event)"=w100, "error IN"=w98, "Frame Number"="FrameCtl", "[IN] Preinitialized Image"=w102, "[IN] AVI Refnum"=w96) -> ("[OUT] Frame"=→"1st Movie (Comparison)":T2)  [unwired: 1 in, 2 out]
        n58 = call "Modify_Image_Histogram-3.vi"("[IN] Parameter"="Gamma", "[IN] Operator"="Operator G Correction", "1 - Origin\n2 - LoG"=u8 1 ("# channel"), "error IN"=w91, "[IN] Image Filtering Settings"=w90, "[IN] LoG Processed Image"=w92) -> ("error OUT"=w83:errorcluster, "[OUT] Image Filtering Settings"=w84:T13, "[OUT] Histogram Modified Image"=→"1st Movie":T2)  [unwired: 2 in, 1 out]
      }
      event "Gray or Binarized?", "FrameCtl2", "Sigma", "Index for thresholding", "Keep Nega-\ntive Values?", "Operator LoG", "Parameter LoG": Value Change {
        w128 = u32 0 items=["Grayscale", "Binary", "Gradient", "Rainbow", "Temperature", "User Defined"] ("Palette:Palette Type")
        w132 = u32 1 items=["Grayscale", "Binary", "Gradient", "Rainbow", "Temperature", "User Defined"] ("Palette:Palette Type")
        w138 = i8 1 ("[IN] Number of event")
        n59 = event-data() -> ()  [unwired: 1 in, 1 out]
        n60 = Decrement(x=w142) -> (x-1=w148:u32)
        n61 = property on="FrameCtl2" class="DigNum (strict)"(error in=w141, "Maximum"=w148, "Minimum"=0.0 ("Data Entry Limits:Minimum")) -> ()  [unwired: 1 in, 2 out]
        n62 = Number To Decimal String(number=w138) -> (decimal integer string=w116:string)  [unwired: 1 in]
        n63 = call "Get_Preinitialized_Images-1.vi"("error IN"=w141, "[IN] Number of event"=w138, "[IN] Images Array"=w140) -> ("error OUT"=w139:errorcluster, "[OUT] Processed Image #1"=w136:T2, "[OUT] Source Image #2"=w119:T2, "[OUT] Source Image #1"=w137:T2)  [unwired: 1 in, 1 out]
        n64 = Not(x="Gray or Binarized?") -> (.not. x?=w150:bool)
        n65 = case shown="False" w150 {
          tunnel: w139 -> [w191 w217]
          tunnel: [w186 w196] -> w122
          tunnel: [w190 w197] -> w123
          tunnel: "Sigma" -> [w164 w201]
          tunnel: "FrameCtl2" -> [w182 w211]
          tunnel: "Index for thresholding" -> [w177 _]
          tunnel: w144 -> [w175 w216]
          tunnel: [w172 w216] -> w143
          tunnel: w117 -> [w181 w210]
          tunnel: w115 -> [w171 w213]
          tunnel: w116 -> [w184 w215]
          tunnel: w137 -> [w183 w212]
          tunnel: w136 -> [w166 w200]
          tunnel: "Keep Nega-\ntive Values?" -> [w163 w203]
          tunnel: "Parameter LoG" -> [w152 w192]
          tunnel: "Operator LoG" -> [w153 w193]
          tunnel: w132 -> [w179 _]
          tunnel: w128 -> [_ w209]
          tunnel: w127 -> [w158 w198]
          tunnel: [w157 w194] -> w126
          frame False {
            n66 = property on="1st Movie Processed" class="ImageControl"(error in=w191, "Palette Type"=w179) -> (error out=w185:errorcluster)  [unwired: 1 in, 1 out]
            n67 = call "Refresh_Image_by_Copying_Fresh_One-1.vi"("[IN] Image Type"=w171, "[IN] Unique ID\n(# of Event)"=w184, "error IN"=w185, "Frame Number"=w182, "[IN] Preinitialized Image"=w183, "[IN] AVI Refnum"=w181) -> ("error OUT"=w168:errorcluster, "[OUT] Frame"=w170:T2)  [unwired: 1 in, 1 out]
            n68 = call "Modify_Image_Histogram-4.vi"("1 - Origin\n2 - LoG"=u8 1 ("# channel"), "error IN"=w168, "[IN] Image Filtering Settings"=w158, "[IN] LoG Processed Image"=w170) -> ("error OUT"=w165:errorcluster, "[OUT] Histogram Modified Image"=w167:T2)  [unwired: 5 in, 1 out]
            n69 = call "Localize_Particles-10.vi"("Keep Nega-\ntive Values?"=w163, "error IN"=w165, "[IN] Sigma"=w164, "[IN] Destination Image"=w166, "[IN] Frame"=w167) -> ("error OUT"=w159:errorcluster, "[OUT] LoG Processed Image"=w162:T2)  [unwired: 3 in, 1 out]
            n70 = call "Modify_Image_Histogram-3.vi"("[IN] Parameter"=w152, "[IN] Operator"=w153, "1 - Origin\n2 - LoG"=u8 2 ("1 - Origin\n2 - LoG"), "error IN"=w159, "[IN] Image Filtering Settings"=w158, "[IN] LoG Processed Image"=w162) -> ("error OUT"=w156:errorcluster, "[OUT] Image Filtering Settings"=w157:T13, "[OUT] Histogram"=w155:T15, "[OUT] Histogram Modified Image"=w154:T2)  [unwired: 2 in]
            n71 = call "Get_Initial_Value_For_Thresholding-1.vi"("[IN] Histogram Graph"=w155, "error IN"=w156) -> ("[OUT] Index of starting \npoint for thresholding"=w178:i32, "[OUT] Minimal index for \nthresholding (negative)"=w189:i32, "[OUT] Maximal index \nfor thresholding"=w188:i32, "error OUT"=w180:errorcluster)
            n72 = property on="Index for thresholding" class="DigNum (strict)"(error in=w180, "Maximum"=w188, "Minimum"=w189) -> (error out=w176:errorcluster)  [unwired: 1 in, 1 out]
            n73 = call "Get_Intensity_Value_For_Thresholding-2.vi"("[IN] Index for \nthresholding"=w177, "error IN"=w176, "[IN] Binarization Set\ntings (Both Channels)"=w175, "[IN] 1 or 2 channel"=u8 1, "[IN] Index of starting \npoint for thresholding"=w178) -> ("error OUT"=w173:errorcluster, "[OUT] Binarization Set\ntings (Both Channels)"=w172:cluster{"MinBin2":sgl, "MaxBin2":sgl}[], "[OUT] For Operator \nBinarization Values"=w174:cluster{"MinBin2":sgl, "MaxBin2":sgl})  [unwired: 1 in]
            n74 = call "IMAQ Threshold"("Replace Value"=sgl 9.0, "error in (no error)"=w173, "Range"=w174, "Image Src"=w154) -> ("error out"=w186:errorcluster, "Image Dst Out"=w190:T2)  [unwired: 6 in]
          }
          frame True {
            n75 = property on="1st Movie Processed" class="ImageControl"(error in=w217, "Palette Type"=w209) -> (error out=w214:errorcluster)  [unwired: 1 in, 1 out]
            n76 = call "Refresh_Image_by_Copying_Fresh_One-1.vi"("[IN] Image Type"=w213, "[IN] Unique ID\n(# of Event)"=w215, "error IN"=w214, "Frame Number"=w211, "[IN] Preinitialized Image"=w212, "[IN] AVI Refnum"=w210) -> ("error OUT"=w208:errorcluster, "[OUT] Frame"=w207:T2)  [unwired: 1 in, 1 out]
            n77 = call "Modify_Image_Histogram-4.vi"("1 - Origin\n2 - LoG"=u8 1 ("# channel"), "error IN"=w208, "[IN] Image Filtering Settings"=w198, "[IN] LoG Processed Image"=w207) -> ("error OUT"=w202:errorcluster, "[OUT] Histogram Modified Image"=w204:T2)  [unwired: 5 in, 1 out]
            n78 = call "Localize_Particles-10.vi"("Keep Nega-\ntive Values?"=w203, "error IN"=w202, "[IN] Sigma"=w201, "[IN] Destination Image"=w200, "[IN] Frame"=w204) -> ("error OUT"=w195:errorcluster, "[OUT] LoG Processed Image"=w199:T2)  [unwired: 3 in, 1 out]
            n79 = call "Modify_Image_Histogram-3.vi"("[IN] Parameter"=w192, "[IN] Operator"=w193, "1 - Origin\n2 - LoG"=u8 2 ("# channel"), "error IN"=w195, "[IN] Image Filtering Settings"=w198, "[IN] LoG Processed Image"=w199) -> ("error OUT"=w196:errorcluster, "[OUT] Image Filtering Settings"=w194:T13, "[OUT] Histogram Modified Image"=w197:T2)  [unwired: 2 in, 1 out]
          }
        }
        "1st Movie Processed" <- w123
        n80 = call "Refresh_Image_by_Copying_Fresh_One-1.vi"("[IN] Image Type"=w115, "[IN] Unique ID\n(# of Event)"=w116, "error IN"=w122, "Frame Number"="FrameCtl2", "[IN] Preinitialized Image"=w119, "[IN] AVI Refnum"=w117) -> ("error OUT"=w120:errorcluster, "[OUT] Frame"=→"1st Movie Original":T2)  [unwired: 1 in, 1 out]
        n81 = call "Modify_Image_Thresholding_Settings-2.vi"("[IN] Image Filtering Settings"=w126, "[IN] Index for thresholding"="Index for thresholding", "[IN] Sigma"="Sigma") -> ("[OUT] Image Filtering Settings"=w114:T13)  [unwired: 6 in]
      }
      event "Try my filters!", "Connectivity", "# Erosion", "Find ALL objects", "Save pics (ex)", "# of Frame": Value Change {
        n82 = event-data() -> ()  [unwired: 1 in, 1 out]
        n83 = Unbundle By Name(w219) -> ("Particle Fil Setups"=w224:T16)
        n84 = Decrement(x=w223) -> (x-1=w255:u32)
        n85 = call "Get_Values_Particle_Filter-1.vi"("Max  Diam"="Max  Diam", "Min  Diam"="Min  Diam") -> ("type of filters\nparticles search"=w241:T17)
        n86 = control-ref of="Detection Progress"() -> (w225:refnum<vi>)
        n87 = property on="# of Frame" class="DigNum (strict)"(error in=w234, "Maximum"=w255, "Minimum"=0.0 ("Data Entry Limits:Minimum")) -> (error out=w247:errorcluster)  [unwired: 1 in, 1 out]
        n88 = call "Merge_Particle_Filter_Setups-1.vi"("[IN] Particle Filter Setups"=w224, "type of filters\nparticles search"=w241, "Connectivity"="Connectivity", "# Erosion"="# Erosion") -> ("[OUT] Particle Filter Setups"=w240:T16)  [unwired: 3 in]
        n89 = property on="Keep Nega-\ntive Values?" class="Bool (strict)"(error in=w247) -> (error out=w226:errorcluster, "Value"=w238:bool)  [unwired: 1 in, 1 out]
        n90 = call "Merge_Localization_Settings_in_Cluster-1.vi"("[IN] Binarization Settings"=w237, "[IN] AVI Refnum"=w228, "[IN] Image Filtering Settings"=w227, "[IN] Image Type"=w236, "[IN] Keep Nega-\ntive Values?"=w238, "[IN] # Channel"=u8 1 ("# Channel"), "[IN] Particle Filter Setups"=w240) -> ("[OUT] Localization Settings"=w218:T8)  [unwired: 4 in]
        n91 = call "Visualize_Results_of_Filtering-1.vi"("[IN] Number of event"=i8 2, "error IN"=w234, "[IN] Localization Settings"=w218, "# Frame"="# of Frame", "[IN] Images Array"=w233) -> ("error OUT"=w229:errorcluster, "[OUT] LoG with Particles"=w230:T2, "[OUT] Binarized Image"=→"1st Filtering":T2)  [unwired: 4 in]
        "Results on 1st Movie" <- w230
        n92 = call "Localization_of_Objects-1.vi"("[IN] Detection Progress"=w225, "[IN] Number of Frames"=w223, "error IN"=w226, "[IN] Find ALL objects"="Find ALL objects", "[IN] Movie Related Values"=w219, "[IN] Localization Settings"=w218) -> ("error OUT"=w222:errorcluster, "[OUT] Movie Related Values"=w221:T11)  [unwired: 4 in]
        n93 = Merge Errors(w229, w222) -> (w248:errorcluster)
        n94 = case shown="True" "Save pics (ex)" {
          tunnel: w248 -> [w257 w259]
          tunnel: [w257 w260] -> w252
          tunnel: w230 -> [_ w258]
          frame False {
          }
          frame True {
            n95 = call "SavePics1.vi"("error IN"=w259, "default name"="Proces_Img2", "Image Dst IN"=w258) -> ("error out"=w260:errorcluster)  [unwired: 1 in]
          }
        }
      }
      event "Tracking Procedure": Value Change {
        n96 = event-data() -> ()  [unwired: 1 in, 1 out]
        n97 = control-ref of="Max angle"() -> (w285:refnum<vi>)
        n98 = control-ref of="Closing gaps"() -> (w287:refnum<vi>)
        n99 = control-ref of="Min TRK L"() -> (w284:refnum<vi>)
        n100 = control-ref of="dR min"() -> (w276:refnum<vi>)
        n101 = control-ref of="dR max"() -> (w275:refnum<vi>)
        n102 = control-ref of="% linearity"() -> (w286:refnum<vi>)
        n103 = call "Buttons_Limits(Tracking_Page)-1.vi"("[IN] dR max"=w275, "[IN] % linearity"=w286, "[IN] dR min"=w276, "[IN] Min TRK L"=w284, "error IN"=w289, "[IN] Number of Frames"=w288, "[IN] Max angle"=w285, "[IN] Closing gaps"=w287) -> ("error OUT"=w268:errorcluster)  [unwired: 3 in]
        n104 = control-ref of="Tracking progress"() -> (w277:refnum<vi>)
        n105 = Bundle("dR min"="dR min", "dR max"="dR max", "Closing gaps"="Closing gaps", "Min TRK L"="Min TRK L", "% linearity"="% linearity", "Max angle"="Max angle", "Tracking progress"=w277) -> (w270:T10)  [unwired: 1 in]
        n106 = call "Tracking_SubVI-5.vi"("[IN] Control Parameters"=w270, "error IN"=w268, "[IN] Before-After Tracks"=w269, "[IN] Movie Values"=w271) -> ("error OUT"=w264:errorcluster, "[OUT] Before-After Tracks"=w265:T12, "[OUT] Obtained Movie Values"=w267:T11, "[OUT] Number of \nRaw Displacements"=→"Raw #":i32)  [unwired: 4 in]
      }
      event "Filter Tracks": Value Change {
        n107 = event-data() -> ()  [unwired: 1 in, 1 out]
        n108 = call "Apply_Filters_to_Tracks-3.vi"("error IN"=w300, "[IN] Control Parameters"=w301, "[IN] Movie Values"=w302) -> ("error OUT"=w296:errorcluster, "[OUT] Filtered Tracks"=w297:T18, "[OUT] # Displ \nafter Filtration"=→"Saved #":i32, "[OUT] Filtered Movie Values"=w298:T11)  [unwired: 4 in, 1 out]
        n109 = control-ref of="Save pictures"() -> (w307:refnum<vi>)
        n110 = control-ref of="Delete Tracs"() -> (w306:refnum<vi>)
        n111 = control-ref of="Raw #"() -> (w310:refnum<vi>)
        n112 = control-ref of="Saved #"() -> (w309:refnum<vi>)
        n113 = control-ref of="Frame"() -> (w308:refnum<vi>)
        n114 = call "Disactivate_Frames_Until_Get_Tracking_Results-1.vi"("Delete Tracs Ref"=w306, "Save pictures Ref"=w307, "error IN"=w296, "Frame Ref"=w308, "Saved #  Ref"=w309, "Raw # Ref"=w310) -> ()  [unwired: 6 in]
        n115 = call "Calculation_Tracks_Statistics-4.vi"("error IN"=w296, "[IN] Tracks Statistics"=w294, "[IN] Filtered Tracks"=w297, "[IN] Movie Values"=w298) -> ("error OUT"=w295:errorcluster, "[OUT] Tracks Statistics"=w293:T14)  [unwired: 6 in]
      }
      event "dR min", "dR max", "Min TRK L", "Max angle", "% linearity": Value Change {
        n116 = event-data() -> ()  [unwired: 1 in, 1 out]
        n117 = property on="dR min" class="DigNum (strict)"(error in=w316) -> ("Value"=w327:dbl)  [unwired: 1 in, 2 out]
        n118 = property on="dR max" class="DigNum (strict)"(error in=w316) -> ("Value"=w321:dbl)  [unwired: 1 in, 2 out]
        n119 = property on="Max angle" class="DigNum (strict)"(error in=w316) -> ("Value"=w315:dbl)  [unwired: 1 in, 2 out]
        n120 = property on="% linearity" class="DigNum (strict)"(error in=w316) -> ("Value"=w317:i32)  [unwired: 1 in, 2 out]
        n121 = property on="Min TRK L" class="DigNum (strict)"(error in=w316) -> ("Value"=w318:i32)  [unwired: 1 in, 2 out]
        n122 = Unbundle(w328) -> ("Closing gaps"=w320:i32, "Tracking progress"=w319:refnum<vi>)  [unwired: 5 out]
        n123 = Bundle(cluster=w328, "dR min"=w327, "dR max"=w321, "Closing gaps"=w320, "Min TRK L"=w318, "% linearity"=w317, "Max angle"=w315, "Tracking progress"=w319) -> (w313:T10)
      }
      event "Show Distributions", "Bins": Value Change {
        n124 = event-data() -> ()  [unwired: 1 in, 1 out]
        n125 = call "Calculation_Statistic_Values-2.vi"("Intervals"="Bins", "[IN] Tracks Statistics"=w341) -> ("[OUT] Representation"=w339:T19)  [unwired: 3 in]
        n126 = Unbundle(w339) -> ("All Instant Vel-s"=→"All Instant Vels":T4, "mean"=→"mean Instant Vel":dbl, "standard deviation"=→"StD Instant":dbl, "All Path Vel-s"=→"All Path Vels":T4, "mean"=→"mean Path Vel":dbl, "standard deviation"=→"StD Path":dbl, "Mean Instan Vel-s"=→"Mean Instant Velocities for Each Track":T4, "Duration of tracks"=→"Duration of Tracks":T4)  [unwired: 4 out]
      }
      event "Frame", "Delete Tracs", "Save pictures": Value Change {
        w356 = i8 3 ("[IN] Number of event")
        n127 = event-data() -> ()  [unwired: 1 in, 1 out]
        n128 = Decrement(x=w373) -> (x-1=w377:u32)
        n129 = property on="Frame" class="DigNum (strict)"(error in=w358, "Maximum"=w377, "Minimum"=0.0 ("Data Entry Limits:Minimum")) -> ()  [unwired: 1 in, 2 out]
        n130 = Unbundle By Name(w379) -> ("Tracks, Coordinates"=w375:T20)
        n131 = call "Visualize_Results_of_Filtering-1.vi"("[IN] Number of event"=w356, "error IN"=w358, "[IN] Localization Settings"=w352, "# Frame"="Frame", "[IN] Images Array"=w351) -> ("error OUT"=w354:errorcluster, "[OUT] LoG with Particles"=w357:T2)  [unwired: 4 in, 1 out]
        n132 = Increment(x=w356) -> (x+1=w355:i8)
        n133 = Unbundle By Name(w375) -> ("(X,Y,dX,dY) NN filtered"=w361:dbl[][], "(X,Y,dX,dY) TH filtered"=w371:dbl[][])
        n134 = call "Visualize_Results_of_Filtering-1.vi"("[IN] Number of event"=w355, "error IN"=w354, "[IN] Localization Settings"=w352, "# Frame"="Frame", "[IN] Images Array"=w351) -> ("error OUT"=w350:errorcluster, "[OUT] LoG with Particles"=w349:T2)  [unwired: 4 in, 1 out]
        n135 = call "Paint_Tracks_on_Frame-1.vi"("Delete \nOverlay?"="Delete Tracs", "[IN] Number of event"=i8 24, "[IN] Images Array"=w351, "error IN"=w350, "# Frame"="Frame", "[IN] #1 Array (X,Y,...)"=w361, "[IN] #1 Processed Image"=w357) -> ("error OUT"=w363:errorcluster, "[OUT] #1 Overlayed Image"=w364:T2)  [unwired: 2 in]
        "1st Filtering (NN)" <- w364
        n136 = call "Paint_Tracks_on_Frame-1.vi"("Delete \nOverlay?"="Delete Tracs", "[IN] Number of event"=i8 21, "[IN] Images Array"=w351, "error IN"=w363, "# Frame"="Frame", "[IN] #1 Array (X,Y,...)"=w371, "[IN] #1 Processed Image"=w349) -> ("error OUT"=w368:errorcluster, "[OUT] #1 Overlayed Image"=w369:T2)  [unwired: 2 in]
        "1st Filtered" <- w369
        n137 = case shown="True" "Save pictures" {
          tunnel: w369 -> [_ w389]
          tunnel: w364 -> [_ w386]
          tunnel: w368 -> [w382 w388]
          tunnel: [w382 w383] -> w380
          frame False {
          }
          frame True {
            n138 = call "SavePics1.vi"("error IN"=w388, "default name"="Track_Img1", "Image Dst IN"=w389) -> ("error out"=w384:errorcluster)  [unwired: 1 in]
            n139 = call "SavePics1.vi"("error IN"=w384, "default name"="Track_Img2", "Image Dst IN"=w386) -> ("error out"=w383:errorcluster)  [unwired: 1 in]
          }
        }
      }
      event "Testing Frame", "Save pics below", "Tracks group", "Save videos \nbelow as *avi": Value Change {
        w408 = i8 5 ("[IN] Number of event")
        n140 = event-data() -> ()  [unwired: 1 in, 1 out]
        n141 = Unbundle(w418) -> ("Before Grouped Tracks"=w409:T21, "After Grouped Tracks"=w404:T21, "Current\nGroup"=w431:i32)
        n142 = Array Size(array=w409) -> (size(s)=w427:i32)
        n143 = call "Get_Info_Before-After_Tracks-1.vi"("[IN] After Tracks"=w404, "[IN] Tracks group"="Tracks group", "[IN] Before Tracks"=w409) -> ("[OUT] Maximal Frame\n(finish point all tracks)"=w425:i32, "[OUT] Min Start Pos"=w424:i32)
        n144 = Decrement(x=w427) -> (x-1=w426:i32)
        n145 = property on="Tracks group" class="DigNum (strict)"(error in=w412, "Maximum"=w426, "Minimum"=0.0 ("Data Entry Limits:Minimum")) -> (error out=w432:errorcluster)  [unwired: 1 in, 1 out]
        n146 = property on="Testing \nFrame" class="DigNum (strict)"(error in=w432, "Maximum"=w425, "Minimum"=w424) -> (error out=w430:errorcluster)  [unwired: 1 in, 1 out]
        n147 = To Unsigned Long Integer(number=w424) -> (unsigned 32bit integer=w423:u32)
        n148 = property on="Tracks \ngroup" class="DigNum (strict)"(error in=w430) -> (error out=w428:errorcluster, "Value"=w417:i32)  [unwired: 1 in, 1 out]
        n149 = in-place {
          in-place-border: w417 -> [w437]
          n150 = in-place-cluster #1(w418) -> ()  [unwired: 1 out]
          n151 = in-place-cluster #1("Current\nGroup"=w437) -> (w416:T12)
        }
        n152 = Equal?(x=w417, y=w431) -> (x = y?=w422:bool)
        n153 = case shown="True" w422 {
          tunnel: w428 -> [w440 w442]
          tunnel: w423 -> [w438 _]
          tunnel: [w439 w442] -> w411
          tunnel: [w438 w441] -> w406
          tunnel: "Testing Frame" -> [_ w441]
          frame False {
            n154 = property on="Testing \nFrame" class="DigNum (strict)"(error in=w440, "Value"=w438) -> (error out=w439:errorcluster)  [unwired: 1 in, 1 out]
          }
          frame True {
          }
        }
        n155 = call "Merge_Grouped_Tracks_Values-1.vi"("[IN] Testing Frame"=w406, "[IN] Tracks group"="Tracks group", "[IN] Grouped Tracks"=w409) -> ("[OUT] Grouped Tracks Values"=w401:T22)  [unwired: 2 in]
        n156 = call "Merge_Grouped_Tracks_Values-1.vi"("[IN] Testing Frame"=w406, "[IN] Tracks group"="Tracks group", "[IN] Grouped Tracks"=w404) -> ("[OUT] Grouped Tracks Values"=w395:T22)  [unwired: 2 in]
        n157 = call "Paint_Tracks_Before-After-4.vi"("[IN] Number of event"=w408, "[IN] Localization Settings"=w396, "[IN] Images Array"=w393, "error IN"=w411, "[IN] Grouped Tracks Values"=w401) -> ("error OUT"=w407:errorcluster, "[OUT] Image with\nDisplacements"=w410:T2)  [unwired: 5 in]
        "Connected and Grouped Tracks" <- w410
        n158 = Increment(x=w408) -> (x+1=w399:i8)
        n159 = call "Paint_Tracks_Before-After-4.vi"("[IN] Number of event"=w399, "[IN] Localization Settings"=w396, "[IN] Images Array"=w393, "error IN"=w407, "[IN] Grouped Tracks Values"=w395) -> ("error OUT"=w402:errorcluster, "[OUT] Image with\nDisplacements"=w403:T2)  [unwired: 5 in]
        "After Resolving Correspondence Problem" <- w403
        n160 = Increment(x=w399) -> (x+1=w392:i8)
        n161 = call "Save_Before-After_Tracks-4.vi"("Save movies?"="Save videos \nbelow as *avi", "[IN] Number of event"=w392, "[IN] Localization Settings"=w396, "[IN] Images Array"=w393, "error IN"=w402, "[IN] FPS"="FPS Gr", "default name"="Tracks_Before_Filt", "[IN] Grouped Tracks Values"=w401) -> ("error OUT"=w398:errorcluster)  [unwired: 3 in]
        n162 = case shown="True" "Save pics below" {
          tunnel: w410 -> [_ w446]
          tunnel: w402 -> [w443 w448]
          tunnel: [w443 w447] -> w429
          tunnel: w403 -> [_ w445]
          frame False {
          }
          frame True {
            n163 = Two Button Dialog(message="1 or 2?", 1:"After" ("F button name (\"Cancel\")"), 2:"Before" ("T button name (\"OK\")")) -> (T button?=w450:bool)
            n164 = case shown="True" w450 {
              tunnel: "Trck_ImgN" ("default name") -> [w455 w460]
              tunnel: w448 -> [w456 w459]
              tunnel: [w453 w458] -> w447
              tunnel: w446 -> [_ w457]
              tunnel: w445 -> [w454 _]
              frame False {
                n165 = call "SavePics1.vi"("error IN"=w456, "default name"=w455, "Image Dst IN"=w454) -> ("error out"=w453:errorcluster)  [unwired: 1 in]
              }
              frame True {
                n166 = call "SavePics1.vi"("error IN"=w459, "default name"=w460, "Image Dst IN"=w457) -> ("error out"=w458:errorcluster)  [unwired: 1 in]
              }
            }
          }
        }
        n167 = Increment(x=w392) -> (x+1=w391:i8)
        n168 = call "Save_Before-After_Tracks-4.vi"("Save movies?"="Save videos \nbelow as *avi", "[IN] Number of event"=w391, "[IN] Localization Settings"=w396, "[IN] Images Array"=w393, "error IN"=w398, "[IN] FPS"="FPS Gr", "default name"="Tracks_After_Filt", "[IN] Grouped Tracks Values"=w395) -> ()  [unwired: 3 in, 1 out]
      }
      event "Save movies": Value Change {
        n169 = event-data() -> ()  [unwired: 1 in, 1 out]
        n170 = Unbundle By Name(w477) -> ("Tracks, Coordinates"=w464:T20)
        n171 = Unbundle By Name(w464) -> ("(X,Y,dX,dY) TH filtered"=w473:dbl[][])
        n172 = call "Save_Tracking_Results_Movie-2.vi"("Save movies"="Save movies", "FPS"="FPS", "# codec"=4, "error IN"=w474, "AVI Refnum"=w471, "default name"="Processed_Movie1", "(X,Y,dX,dY)"=w473) -> ("error out"=w468:errorcluster)  [unwired: 4 in]
      }
      event "Save All Instant Vels", "Save Path Velocities", "Save Mean Velocities", "Save Duration of Tracks", "Save Tracks in Columns (x,y,dx,dy)": Value Change {
        n173 = event-data() -> ()  [unwired: 1 in, 1 out]
        n174 = call "Save_Various_Calculated_Vals_1.vi"("[IN] Save Tracks in Columns"="Save Tracks in Columns (x,y,dx,dy)", "[IN] Save Mean Vels for Tracks"="Save Mean Velocities", "[IN] Save Track Durations"="Save Duration of Tracks", "[IN] Save All Path Velocities"="Save Path Velocities", "error IN"=w486, "[IN] Statistics"=w488, "[IN] Save All Instant Velocities"="Save All Instant Vels", "[IN] File Path with Movie"=w485) -> ("error OUT"=w487:errorcluster)  [unwired: 3 in]
      }
      event "STOP Program": Value Change {
        n175 = event-data() -> ()  [unwired: 1 in, 1 out]
        n176 = Index Array(array=w507, index=0) -> (element=w503:T2)
        n177 = call "IMAQ AVI2 Close"("error in (no error)"=w505, "AVI Refnum"=w506) -> ("error out"=w502:errorcluster)  [unwired: 9 in]
        n178 = Request Deallocation("STOP Program") -> ()
        n179 = call "IMAQ Dispose"("All Images? (No)"=TRUE, "Image"=w503, "error in (no error)"=w502) -> ("error out"=w501:errorcluster)  [unwired: 3 in]
      }
      event Timeout {
        n180 = event-data() -> ()  [unwired: 1 in, 1 out]
      }
    }
    "error out" <- w70
    n181 = Unbundle(w70) -> ("code"=w77:i32, "source"=w76:string)  [unwired: 1 out]
    n182 = call <vilib>:"Simple Error Handler.vi"("error code (no error:0)"=w77, "error source (\" \")"=w76, "error in (no error)"=w70) -> ()  [unwired: 2 in, 5 out]
  }
